vi "Find Average Center.vi"(5 "Position":i32, 7 "Tray Number":i32, 8 "Assembly Type":string, 9 "XYZTheta":dbl[](array[numeric]), 10 "Sensor Thickness":dbl, 11 "Gantry In":refnum<k24>) -> (1 "XYZTheta":dbl[](array[numeric]) format="%.6g", 3 "Gantry Out":refnum<k24>)   [LabVIEW 2021, in "Component Tray.lvclass"]
uses:
  Component Tray.lvclass
  Find Component.ctl
  Controller/Camera/Machine Vision.ctl
  C:/Program Files (x86)/Aerotech/A3200/LabVIEW/2010/Bin/Aerotech.A3200.dll
  Program Files (x86)/Aerotech/A3200/LabVIEW/2010/Bin/Aerotech.A3200.dll
  Controller/Camera/Camera settings.ctl
  <vilib>/vision/Pattern Matching.llb/IMAQ Pattern Match Advanced Options.ctl
  Controller/Camera/Edmund Optics/Edmund Optics.lvclass
  C:/Users/HEP/Documents/GitHub/Gantry/UCSB-Gantry-HEP-main/Classes/Controller/Camera/Camera.lvclass
  Controller/Camera/Camera.lvclass
  Controller/Motion/A3200/A3200.lvclass
  Controller/Motion/Motion.lvclass
  <vilib>/vision/NI_Vision_Development_Module.lvlib
  <vilib>/vision/Image Controls.llb/IMAQ Image.ctl
panel:
  in  "Algorithm":i32(ring)=2 items=["All", "Low Discrepancy Sampling", "Grayscale Value Pyramid", "Gradients Pyramid"]
  in  "Parameters":T1={"Number of Matches Requested"=1, "Minimum Match Score"=800.0, "Angle Ranges"=[]}
  in  "ROI Descriptor":T2 {"Contours"."Type" items=["No Selection", "Point", "Line", "Rectangle", "Oval", "Polygon", "Freehand Region", "Annulus", "Unused2", "Unused3", "Broken Line", "Freehand Line", "Rotated Rectangle"]}
  in  "Advanced Options":cluster{"Item":T3, "Value":dbl}[](array[cluster]) {"Item" items=["LD Sampling - Minimum Constrast"=0, "LD Sampling - Enable Subpixel Accuracy"=1, "LD Sampling - Search Strategy"=2, "LD Sampling - Subpixel Iterations"=3, "LD Sampling - Subpixel Tolerance"=4, "LD Sampling - Initial Match List Length"=5, "LD Sampling - Match List Reduction Factor"=6, "LD Sampling - Initial Step Size"=7, "LD Sampling - Intermediate Angular Accuracy"=8, "-"=9, "Pyramid - Max Pyramid Level"=100, "Pyramid - Minimum Contrast"=102, "Pyramid - Enable Subpixel Accuracy"=103, "Pyramid - Subpixel Iterations"=104, "Pyramid - Subpixel Tolerance"=105, "Pyramid - Initial Match List Length"=106, "Pyramid - Match List Reduction Factor"=107, "Pyramid - Intermediate Angular Accuracy"=108, "Pyramid - Process Border Matches"=109, "Pyramid - Min Match Separation Distance"=111, "Pyramid - Min Match Separation Angle"=112, "Pyramid - Max Match Overlap"=113, "Pyramid - Max Cache in MB"=114, "Pyramid - Clear Cache"=115, "Pyramid - Enable Accurate Score Computation"=116, "Pyramid - Interpolation Method For Score Computation"=117, "Pyramid - Enable Target To Template Score"=118, "-"=119, "Enable Defect Map"=200]}
  out "Array":i32[](array[numeric])
  out "Checking Sensor ID":bool
  out "All Matches XY":sgl[][](array[numeric])
  out "Match found?":bool
  in  "Focus":bool
  out "Gantry":dbl[](array[numeric]) format="%.6g"
  out "Sum":dbl[](array[numeric]) format="%.6g"
  in  "Machine Vision":T4
  out "Radius (Real-World)":dbl
  out "Standard Variation":sgl
  out "Maximal Value":sgl
  out "Average Strength":dbl
  out "Instructions":string
  out "Camera":dbl[](array[numeric])
  out "Image":T5(plugin-control)
  in  "Enter Manual Mode":bool
  out "Manual Mode On":bool
  in  "Auto Submit":bool
  out "Tray and Position":string
  out "Sensor ID":picture[](array[picture])
  out "Sensor ID":string
  out "predicted fiducials":dbl[][](array[numeric])
  out "Current Z High Speed":dbl
  out "Current XY High Speed":dbl
  out "current Z low speed":dbl
  out "current XY speed":dbl
  in  "Z high":dbl=12.5
  in  "XY high":dbl=50.0
  in  "Z low":dbl=0.05
  in  "XY low":dbl=0.1
  in  "Predict fiducials":bool
  out "Low Speed":bool
  out "X":bool
  out "Y":bool
  out "Z":bool
  out "High Speed":bool
  in  "Go to CH191/FD5":bool
  in  "Go to CH197/FD4":bool
  out "Program Done?":bool
  out "Sensor ID Location":dbl[](array[numeric])
  in  "Go to Sensor ID":bool
  out "CH1 XYZ":dbl[](array[numeric])
  out "CH1 correct?":bool
  in  "Go to CH1":bool
  out "All fiducials recorded":bool
  in  "Override camera presets":bool
  in  "Camera settings":T6={"Gamma"=1.6, "Gain"=0, "Sharpness"=0, "Contrast"=0.0, "Exposure"=0.0078125} {"Exposure" min=0.000244140625 max=0.5 scale=0.0002..0.5; "Contrast" min=0.0 max=1.0 scale=0.001..1.0; "Sharpness" min=0 max=2 step=1 scale=0.0..2.0; "Gain" min=0 max=100 step=1 scale=0.1..100.0; "Gamma" min=0.01 max=10.0 scale=0.01..10.0}
  out "CH197/FD4 XYZ":dbl[](array[numeric]) format="%.6g"
  out "CH8/FD2 XYZ":dbl[](array[numeric]) format="%.6g"
  out "CH191/FD5 XYZ":dbl[](array[numeric]) format="%.6g"
  out "CH1/FD1 XYZ":dbl[](array[numeric]) format="%.6g"
  in  "Record CH8/FD2":bool
  in  "Record CH197/FD4":bool
  in  "Record CH191/FD5":bool
  in  "Record CH1/FD1":bool
  in  "Go to CH8/FD2":bool
  in  "Go to CH1/FD1":bool
  in  "Joystick":bool
  in  "Go to Center":bool
  in  "Component":T7
  in  "Stop Program":bool
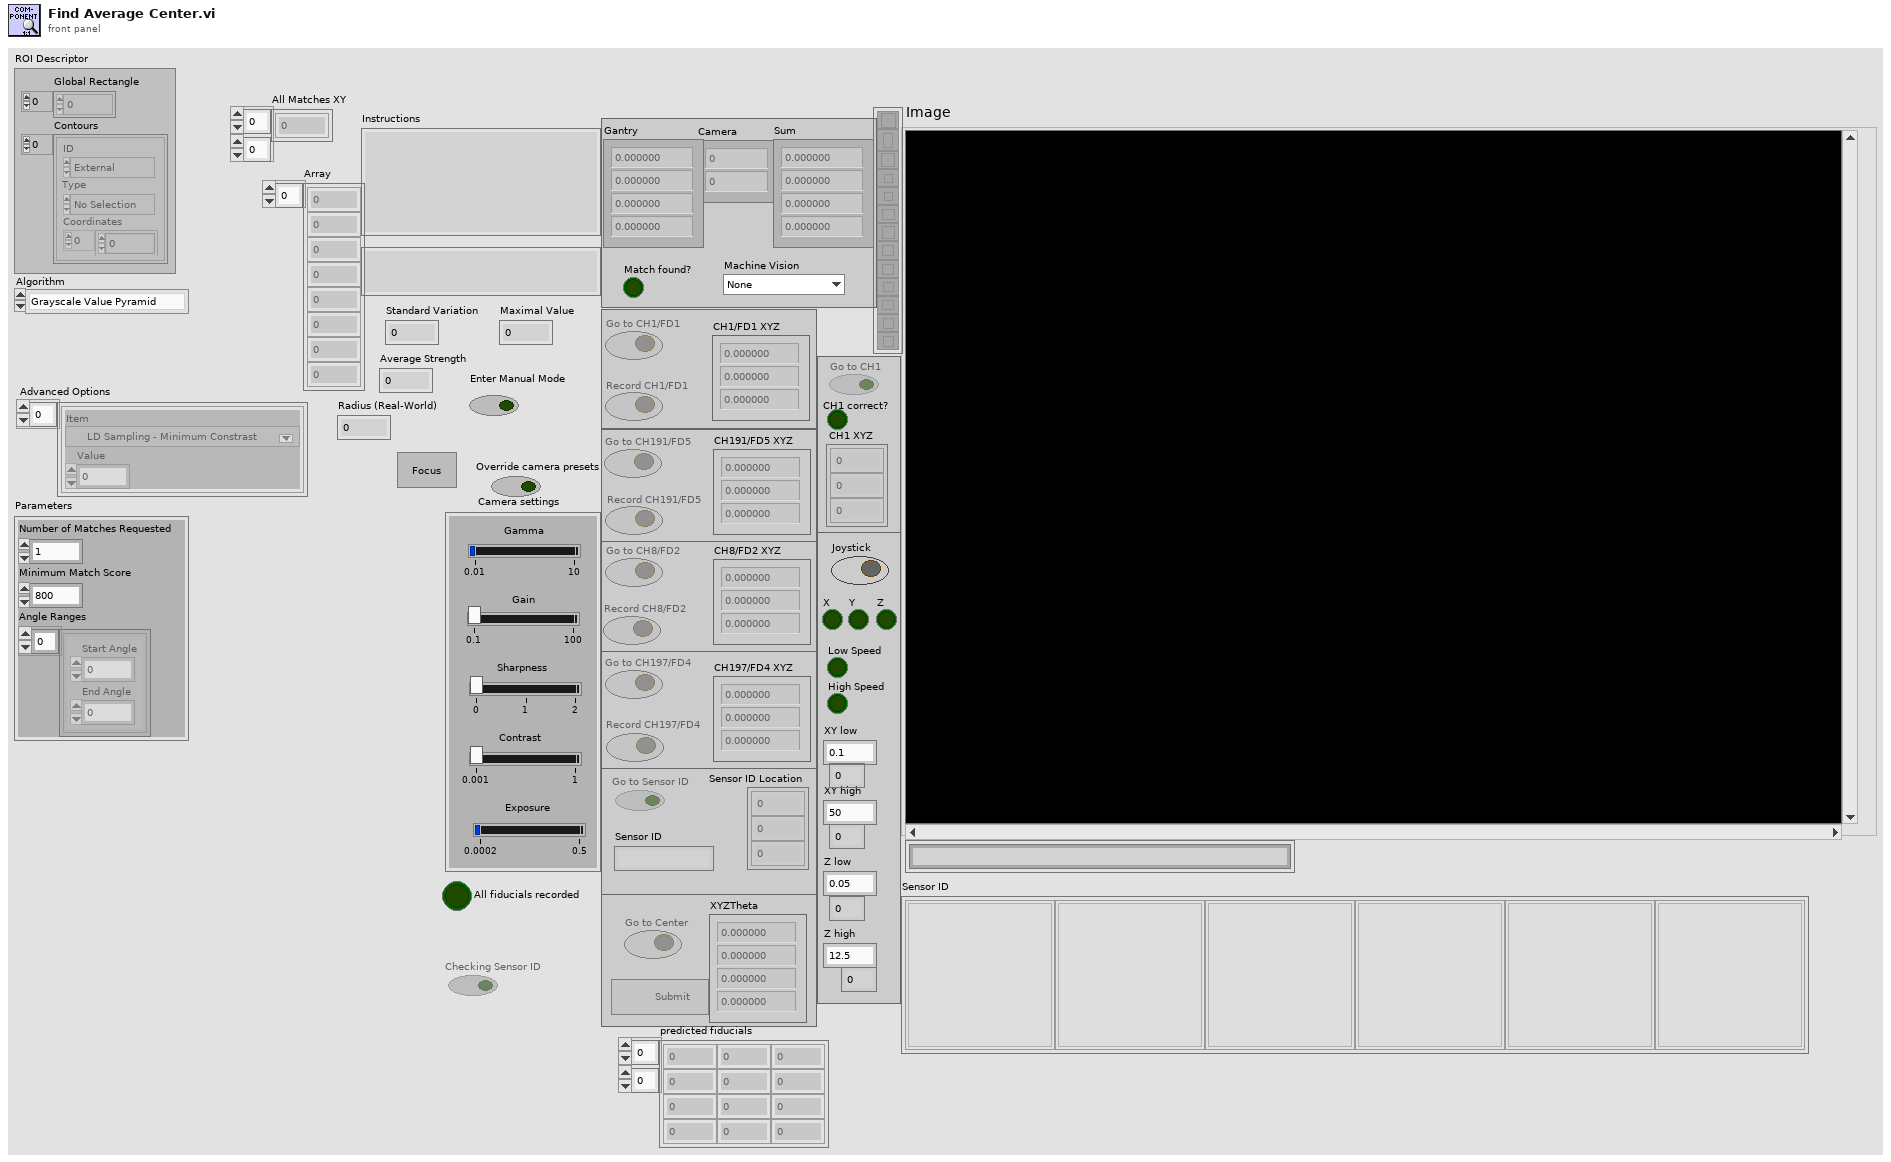
[diagram p1: front panel]
types:
  T1 = cluster{"Number of Matches Requested":i32, "Minimum Match Score":sgl, "Angle Ranges":cluster{"Start Angle":sgl, "End Angle":sgl}[]}
  T2 = typedef "ROI Descriptor" = cluster{"Global Rectangle":i32[], "Contours":cluster{"ID":enum32{"External", "Internal"}, "Type":u32, "Coordinates":i32[]}[]}
  T3 = typedef "IMAQ Pattern Match Advanced Options.ctl" = u16
  T4 = typedef "Camera.lvclass/Machine Vision.ctl" = enum16{"None", "Assembly Tray Circle", "Assembly Tray Fiducial", "Partial Hexaboard", "sensor edge init", "HB edge init", "sensor edge pos1", "sensor edge pos2", "HB edge pos1", "HB edge pos2", "Sensor CH1-2", "HB CH1", "HB CH2", "V3 Sensor Circle", "Hexaboard Circle", "sensor CH1 check", "HB CH1 check ", "sensor ID"}
  T5 = typedef "IMAQ Image.ctl" = refnum<image>
  T6 = typedef "Camera.lvclass/Camera settings.ctl" = cluster{"Gamma":dbl, "Gain":i64, "Sharpness":i64, "Contrast":dbl, "Exposure":dbl}
  T7 = typedef "Component Tray.lvclass/Find Component.ctl" = cluster{"New Fiducials":dbl[], "Past Fiducials":dbl[][], "XYZTheta":dbl[], "Fiducials Path":path, "Position":i32, "CH1 Location":dbl[], "Sensor ID Location":dbl[], "initial rotation":dbl[], "CH2 location":dbl[], "max std variation":dbl, "max strength":dbl, "CH2 pattern matching":T4, "Fiducial Circle":T4, "Get Edge":T4, "Pos multiplier":dbl, "time to wait":u32, "fiducial to edge":dbl, "Protomodule?":bool, "Assembly Type":string, "CH1 to CH2":dbl, "Tray Number":string, "fiducial radius":dbl, "4 fiducials?":bool, "CH1 check":T4, "Edge Scan":T4, "CH1 pattern matching":T4, "Sensor Thickness":dbl, "Previous Avgs":dbl[][], "avg value count":dbl[]}
  T8 = enum8{"Enabled", "Disabled", "Disabled and Grayed Out"}
  T9 = enum16{"None", "Assembly Tray Circle", "Assembly Tray Fiducial", "Partial Hexaboard", "sensor edge init", "HB edge init", "sensor edge pos1", "sensor edge pos2", "HB edge pos1", "HB edge pos2", "Sensor CH1-2", "HB CH1", "HB CH2", "V3 Sensor Circle", "Hexaboard Circle", "sensor CH1 check", "HB CH1 check "}
  T10 = cluster{"Average Strength":dbl, "Radius (Real-World)":dbl, "Match found?":bool, "initial angle":sgl, "Global Report":cluster{"Mean Value":sgl, "Standard Variation":sgl, "Minimal Value":sgl, "Maximal Value":sgl, "Area (calibrated)":sgl, "Area (pixels)":u32, "%":sgl, "Calibration Valid":bool}}
  T11 = typedef "IMAQ GM Match Report.ctl" = cluster{"Position":cluster{"x":sgl, "y":sgl}, "Angle":sgl, "Scale":sgl, "Score":sgl, "Bounding Box":cluster{"x":sgl, "y":sgl}[], "Contrast Reversed":bool, "Occlusion %":sgl, "Template Target Curve Score":sgl, "Target Template Curve Score":sgl, "Correlation Score":sgl}
  T12 = cluster{"Mean Value":sgl, "Standard Variation":sgl, "Minimal Value":sgl, "Maximal Value":sgl, "Area (calibrated)":sgl, "Area (pixels)":u32, "%":sgl, "Calibration Valid":bool}
  T13 = cluster{"left":i16, "top":i16, "right":i16, "bottom":i16}
  T14 = typedef "File Paths.ctl" = cluster{"Glue Pattern Folder":path, "Carrier Tray Folder":path, "Pick Up Tool Fixture Folder":path, "Components Folder":path, "Bellows Tool Offset.txt":path, "Pick Up Tool Offset.txt":path, "Dispense Tip Offset.txt":path, "Log Files":path, "Gantry Assembly Map.txt":path, "Syringe and offset map.txt":path, "Controllers Folder":path, "Local dbase config":path}
  T15 = typedef "imagedata.ctl" = cluster{"image type":i32, "image depth":i32, "image":u8[], "mask":u8[], "colors":u32[], "Rectangle":cluster{"left":i16, "top":i16, "right":i16, "bottom":i16}}
  T16 = cluster{"left":dbl, "top":dbl, "right":dbl, "bottom":dbl}
  T17 = cluster{"Position":cluster{"x":sgl, "y":sgl}, "Angle":sgl, "Scale":sgl, "Score":sgl, "Bounding Box":cluster{"x":sgl, "y":sgl}[]}[]
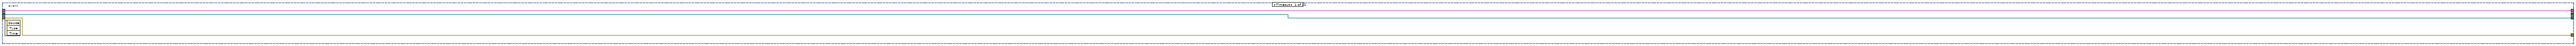
[diagram p3: hidden frame]
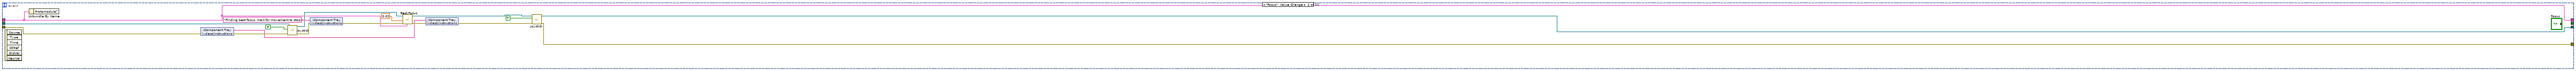
[diagram p4: hidden frame]
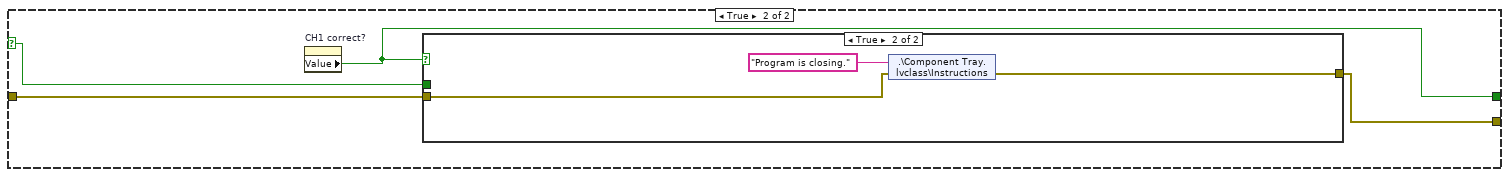
[diagram p5: hidden frame]
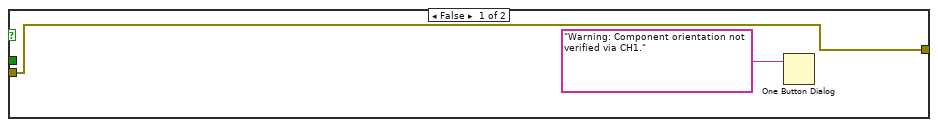
[diagram p6: hidden frame]
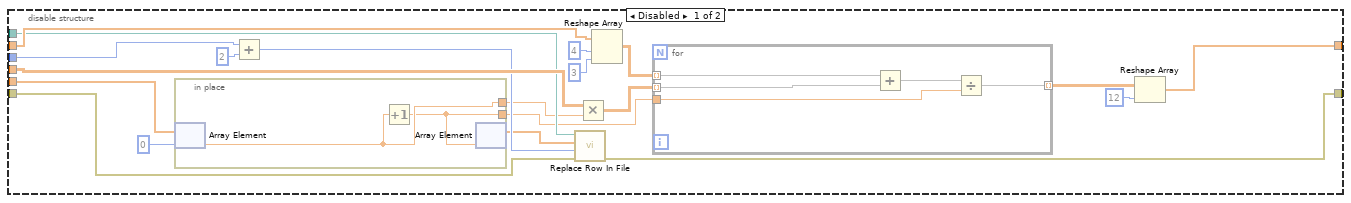
[diagram p8: hidden frame]
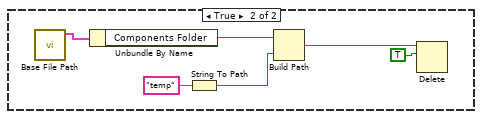
[diagram p9: hidden frame]
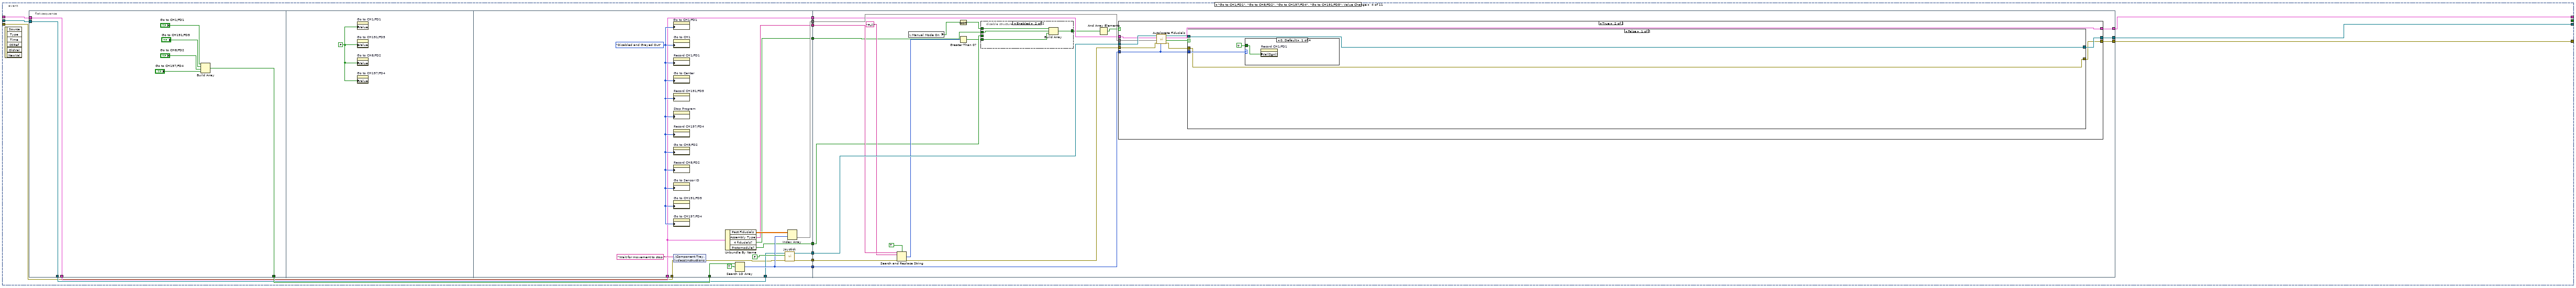
[diagram p10: hidden frame]
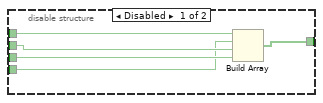
[diagram p11: hidden frame]
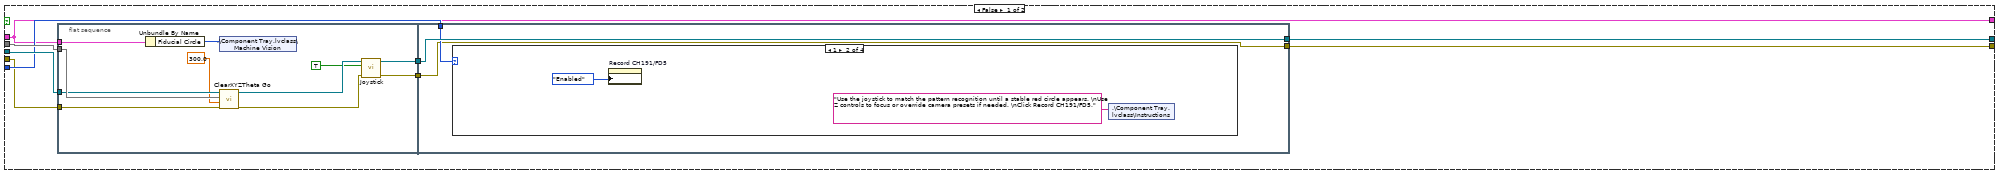
[diagram p12: hidden frame]
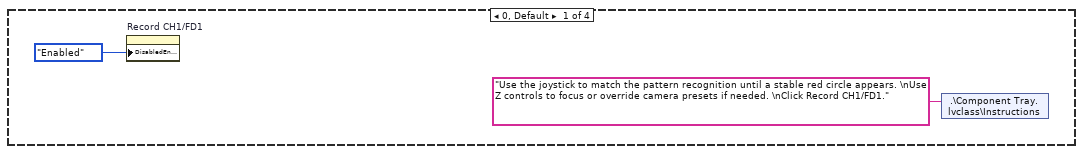
[diagram p13: hidden frame]
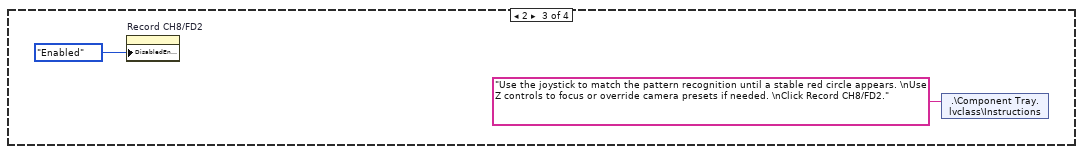
[diagram p14: hidden frame]
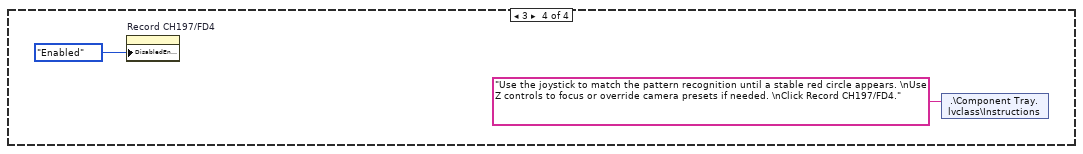
[diagram p15: hidden frame]
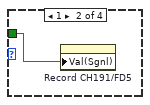
[diagram p16: hidden frame]
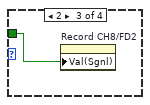
[diagram p17: hidden frame]
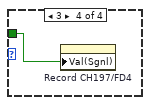
[diagram p18: hidden frame]
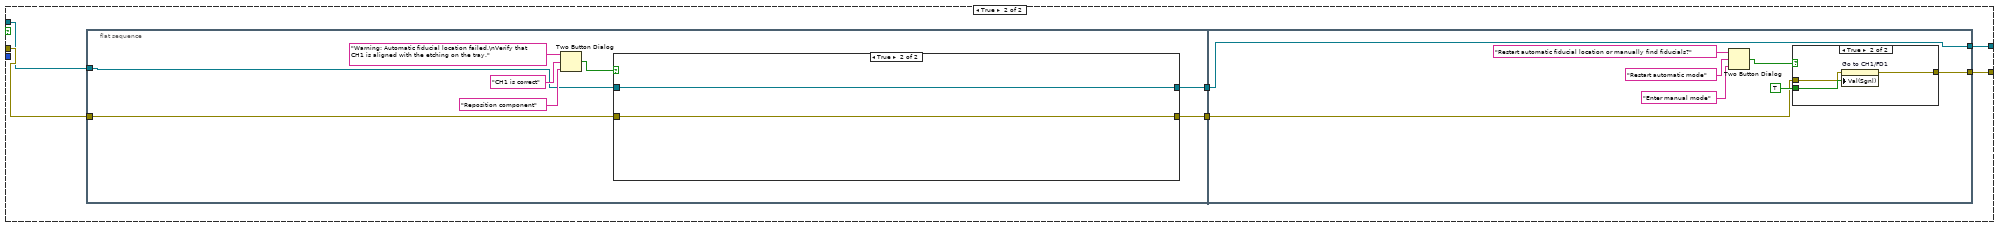
[diagram p19: hidden frame]
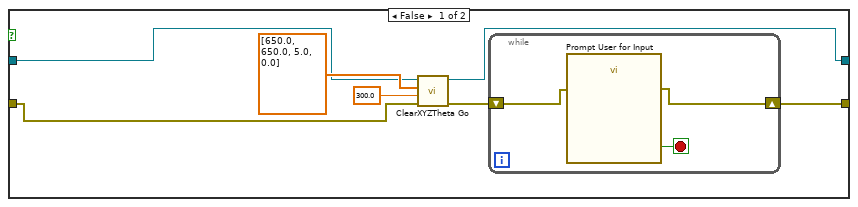
[diagram p20: hidden frame]
diagram:
  n1 = flat-sequence {
    tunnel: [w20] -> w13
    tunnel: [w22] -> w11
    tunnel: ["Gantry In"] -> w9
    tunnel: ["Position"] -> w8
    tunnel: [w28] -> w6
    tunnel: w13 -> [w28]
    tunnel: [w27] -> w5
    tunnel: w11 -> [w27]
    tunnel: [w26] -> w4
    tunnel: w9 -> [w26]
    tunnel: [w25] -> w3
    tunnel: w8 -> [w25]
    tunnel: [w24] -> w1
    tunnel: [w34] -> w12
    tunnel: w6 -> [w34]
    tunnel: w5 -> [w37]
    tunnel: [w37] -> w10
    tunnel: [w36] -> w2
    tunnel: w4 -> [w36]
    tunnel: [w35] -> w7
    tunnel: w3 -> [w35]
    frame #0 {
      w22 = refnum<class "Edmund Optics.lvclass"> refnum  # Edmund Optics.lvclass
      (unwired) 1 ("y")
      n2 = call "Find Average Center Setup.vi"("Sensor Thickness"="Sensor Thickness", "Assembly Type"="Assembly Type", "Position"="Position", "Tray Number"="Tray Number", "XYZTheta"="XYZTheta", "Component"="Component") -> ("output cluster"=w20:T7)  [unwired: 5 in]
    }
    frame #1 {
      n3 = control-ref of="This VI"() -> (w29:refnum<vi>)
      n4 = invoke class="VI" method="Default Vals.Reinit All"(reference=w29) -> (error out=w24:errorcluster)  [unwired: 2 in, 2 out]
    }
    frame #2 {
      n5 = Unbundle By Name(w34) -> ("4 fiducials?"=w30:bool)
      n6 = Select(t=T8."Enabled" ("Disabled"), s=w30, f=T8."Disabled and Grayed Out" ("Disabled")) -> (s? t:f=w31:T8)
      n7 = property on="CH197/FD4 XYZ" class="Arr (strict)"("DisabledEnum"=w31) -> ()  [unwired: 2 in, 2 out]
      n8 = property on="Record CH191/FD5" class="Bool (strict)"("DisabledEnum"=w31) -> ()  [unwired: 2 in, 2 out]
      n9 = property on="Predict fiducials" class="Bool (strict)"("DisabledEnum"=w31) -> ()  [unwired: 2 in, 2 out]
      n10 = property on="Record CH197/FD4" class="Bool (strict)"("DisabledEnum"=w31) -> ()  [unwired: 2 in, 2 out]
      n11 = property on="Go to CH197/FD4" class="Bool (strict)"("DisabledEnum"=w31) -> ()  [unwired: 2 in, 2 out]
      n12 = property on="CH191/FD5 XYZ" class="Arr (strict)"("DisabledEnum"=w31) -> ()  [unwired: 2 in, 2 out]
      n13 = property on="Go to CH191/FD5" class="Bool (strict)"("DisabledEnum"=w31) -> ()  [unwired: 2 in, 2 out]
    }
  }
  n14 = while {
    shift-right: [w62] -> _
    shift-left: w10 -> [w64]
    shift-right: [w45] -> _
    shift-left: w2 -> [w47]
    i -> [w59]
    stop <- w43 stop-if-true
    n15 = in-place {
      in-place-border: [w90] -> w46
      in-place-border: w47 -> [w72]
      # "Joystck Status"
      n16 = call "Get Joytick Status.vi"("Gantry In"=w72) -> ("JoystickLowSpeedActive"=w94:bool, "Joystick Status"=w95:bool[], "Gantry Out"=w91:refnum<k24>, "High Speeds"=w79:dbl[], "Low Speeds"=w78:dbl[])  [unwired: 5 in, 1 out]
      n17 = Build Array("XY low", "XY low", "XY low", "Z low") -> (w85:dbl[])
      n18 = Build Array("XY high", "XY high", "XY high", "Z high") -> (w84:dbl[])
      n19 = call "Set Joystick Speed.vi"("High Speed Inputs"=w84, "Low Speed Inputs"=w85, "Gantry"=w91) -> ("Controller Out"=w90:refnum<k24>)  [unwired: 7 in, 1 out]
      n20 = Or Array Elements(Boolean array=w95) -> (logical OR=w92:bool)
      n21 = Not(x=w94) -> (.not. x?=w93:bool)
      n22 = Index Array(array=w79) -> (element #1=→"Current XY High Speed":dbl, element #3=→"Current Z High Speed":dbl)  [unwired: 3 in, 1 out]
      n23 = Index Array(array=w78) -> (element #1=→"current XY speed":dbl, element #3=→"current Z low speed":dbl)  [unwired: 3 in, 1 out]
      n24 = Index Array(array=w95) -> (element #1=→"X":bool, element #2=→"Y":bool, element #3=→"Z":bool)  [unwired: 3 in]
      n25 = And(x=w93, y=w92) -> (x .and. y?=→"High Speed":bool)
      n26 = And(x=w92, y=w94) -> (x .and. y?=→"Low Speed":bool)
    }
    n27 = local read "Checking Sensor ID"() -> (w38:bool)
    n28 = shared-variable ".\\Component Tray.lvclass\\Instructions"() -> (→"Instructions":string)  [unwired: 1 in, 1 out]
    n29 = property on="Manual Mode On" class="Bool (strict)"() -> ("Value"=w40:bool)  [unwired: 2 in, 2 out]
    n30 = shared-variable ".\\Component Tray.lvclass\\Manual Mode"("Enter Manual Mode") -> ()  [unwired: 1 in, 1 out]
    n31 = Or(x=w40, y=w38) -> (x .or. y?=w39:bool)
    n32 = case shown="True" w39 {
      tunnel: [w96 "Machine Vision"] -> w48
      frame False {
        n33 = shared-variable ".\\Component Tray.lvclass\\Machine Vision"() -> (w96:T9)  [unwired: 1 in, 1 out]
      }
      frame True {
      }
    }
    n34 = local read "Program Done?"() -> (w43:bool)
    n35 = Equal To 0?(x=w59) -> (x = 0?=w58:bool)
    n36 = call "Camera.vi"("Camera in"=w64, "Stop"=w43, "Machine Vision"=w48, "Camera settings"="Camera settings", "Loop 0"=w58, "Override presets"="Override camera presets") -> ("All Matches XY"=→"All Matches XY":sgl[][], "Camera out"=w62:refnum<class "Edmund Optics.lvclass">, "output cluster"=w57:T10, "pattern matching"=w50:T11, "Image"=→"Image":T5, "Camera"=w42:dbl[])  [unwired: 6 in, 2 out]
    "Camera" <- w42
    n37 = Unbundle By Name(w57) -> ("Average Strength"=w56:dbl, "Radius (Real-World)"=w55:dbl, "Match found?"=w54:bool, "Global Report"=w53:T12)
    "Average Strength" <- w56
    "Radius (Real-World)" <- w55
    "Match found?" <- w54
    n38 = shared-variable ".\\Component Tray.lvclass\\pattern matching"(w50) -> ()  [unwired: 1 in, 1 out]
    n39 = shared-variable ".\\Component Tray.lvclass\\Camera"(w42) -> ()  [unwired: 1 in, 1 out]
    n40 = in-place {
      in-place-border: w46 -> [w67]
      in-place-border: [w66] -> w45
      in-place-border: w42 -> [w65]
      # "Current Position"
      n41 = call "Get Current Position.vi"("Gantry In"=w67) -> ("XYZTheta Out"=w70:dbl[], "Gantry Out"=w66:refnum<k24>)  [unwired: 8 in, 1 out]
      "Gantry" <- w70
      n42 = Reshape Array(w65, 4 ("dimension size")) -> (w69:dbl[])
      n43 = Add(x=w70, y=w69) -> (x+y=→"Sum":dbl[])
    }
    n44 = shared-variable ".\\Component Tray.lvclass\\Average Strength"(w56) -> ()  [unwired: 1 in, 1 out]
    n45 = shared-variable ".\\Component Tray.lvclass\\Radius (Real-World)"(w55) -> ()  [unwired: 1 in, 1 out]
    n46 = shared-variable ".\\Component Tray.lvclass\\Match found?"(w54) -> ()  [unwired: 1 in, 1 out]
    n47 = Unbundle By Name(w53) -> ("Standard Variation"=w52:sgl, "Maximal Value"=w51:sgl)
    "Maximal Value" <- w51
    "Standard Variation" <- w52
    n48 = shared-variable ".\\Component Tray.lvclass\\Standard Variation"(w52) -> ()  [unwired: 1 in, 1 out]
    n49 = shared-variable ".\\Component Tray.lvclass\\Maximal Value"(w51) -> ()  [unwired: 1 in, 1 out]
  }
  n50 = while {
    shift-right: [w107] -> _
    shift-left: w12 -> [w100]
    shift-right: [w105] -> w14
    shift-left: w2 -> [w106]
    tunnel: w7 -> [w101]
    shift-right: [w98] -> _
    shift-left: w1 -> [w99]
    i -> [w104]
    stop <- w108 stop-if-true
    n51 = event shown="[2] \"Stop Program\", \"Auto Submit\": Value Change" {
      selector: _ -> [_ _ _ _ _ _ _ _ _ _ _]
      dyn-events: _ -> [_ _ _ _ _ _ _ _ _ _ _]
      timeout: _ -> [_ _ _ _ _ _ _ _ _ _ _]
      tunnel: [_ _ w147 _ _ _ _ _ _ _ _] -> w108
      tunnel: w100 -> [w126 w127 w151 w233 w384 w464 w491 w499 w541 w669 w689]
      tunnel: [w126 w127 w151 w229 w391 w463 w491 w499 w541 w669 w689] -> w107
      tunnel: w106 -> [w125 w134 w152 w237 w407 w468 w490 w498 w547 w671 w688]
      tunnel: [w125 w131 w150 w231 w385 w468 w488 w496 w545 w671 w687] -> w105
      tunnel: w99 -> [w124 w138 w144 w223 w390 w461 w487 w494 w537 w666 w685]
      tunnel: [w124 w128 w145 w221 w388 w461 w486 w492 w535 w666 w684] -> w98
      event Timeout {
        n52 = event-data() -> ()  [unwired: 1 in, 3 out]
      }
      event "Focus": Value Change {
        n53 = event-data() -> ()  [unwired: 1 in, 6 out]
        n54 = Unbundle By Name(w127) -> ()  [unwired: 1 out]
        n55 = shared-variable ".\\Component Tray.lvclass\\Instructions"(error in=w138) -> (w140:string, error out=w136:errorcluster)
        n56 = call "Joystick.vi"("error in (no error)"=w136, "Joystick"=FALSE, "Gantry In"=w134) -> ("error out"=w135:errorcluster, "Gantry Out"=w133:refnum<k24>)  [unwired: 7 in]
        n57 = shared-variable ".\\Component Tray.lvclass\\Instructions"("Finding best focus. Wait for movement to stop." ("Instructions"), error in=w135) -> (error out=w142:errorcluster)
        n58 = call "Best Focus.vi"("Component"=w127, "error in (no error)"=w142, "Inc by"=0.02, "Gantry In"=w133) -> ("error out"=w141:errorcluster, "Gantry Out"=w130:refnum<k24>)  [unwired: 4 in, 2 out]
        n59 = shared-variable ".\\Component Tray.lvclass\\Instructions"(w140, error in=w141) -> (error out=w129:errorcluster)
        n60 = call "Joystick.vi"("error in (no error)"=w129, "Joystick"=TRUE, "Gantry In"=w130) -> ("error out"=w128:errorcluster, "Gantry Out"=w131:refnum<k24>)  [unwired: 7 in]
      }
      event "Stop Program", "Auto Submit": Value Change {
        n61 = event-data() -> ()  [unwired: 1 in, 6 out]
        n62 = flat-sequence {
          frame #0 {
          }
          frame #1 {
            n63 = property on="Auto Submit" class="Bool (strict)"("Value"=FALSE ("Auto Submit")) -> ()  [unwired: 2 in, 2 out]
          }
        }
        n64 = property on="All fiducials recorded" class="Bool (strict)"() -> ("Value"=w149:bool)  [unwired: 2 in, 2 out]
        n65 = case shown="False" w149 {
          selector: w149 -> [w154 w159]
          tunnel: [w154 w158] -> w148
          tunnel: [w153 w157] -> w146
          tunnel: w144 -> [w153 w156]
          frame False {
            n66 = One Button Dialog(message="Warning: At least one fiducial not recorded.") -> ()  [unwired: 1 in, 1 out]
          }
          frame True {
            n67 = property on="CH1 correct?" class="Bool (strict)"() -> ("Value"=w158:bool)  [unwired: 2 in, 2 out]
            n68 = case shown="True" w158 {
              tunnel: w159 -> [_ _]
              tunnel: w156 -> [w160 w163]
              tunnel: [w160 w162] -> w157
              frame False {
                n69 = One Button Dialog(message="Warning: Component orientation not verified via CH1.") -> ()  [unwired: 1 in, 1 out]
              }
              frame True {
                n70 = shared-variable ".\\Component Tray.lvclass\\Instructions"("Program is closing." ("Instructions"), error in=w163) -> (error out=w162:errorcluster)
              }
            }
          }
        }
        n71 = case shown="True" w148 {
          selector: w148 -> [w167 w185]
          tunnel: w152 -> [w168 w184]
          tunnel: w151 -> [_ w182]
          tunnel: [w168 w183] -> w150
          tunnel: [w167 w185] -> w147
          tunnel: w146 -> [w166 w173]
          tunnel: [w166 w170] -> w145
          frame False {
          }
          frame True {
            n72 = Unbundle By Name(w182) -> ("Fiducials Path"=w175:path, "New Fiducials"=w177:dbl[], "Position"=w174:i32, "Protomodule?"=w181:bool, "Previous Avgs"=w178:dbl[][], "avg value count"=w169:dbl[])
            n73 = call "Joystick.vi"("error in (no error)"=w173, "Joystick"=FALSE, "Gantry In"=w184) -> ("error out"=w172:errorcluster, "Gantry Out"=w183:refnum<k24>)  [unwired: 7 in]
            n74 = case shown="False" w181 {
              frame False {
              }
              frame True {
                n75 = call "Base File Path.vi"() -> ("Paths Out"=w219:T14)  [unwired: 11 in]
                n76 = Unbundle By Name(w219) -> ("Components Folder"=w217:path)
                n77 = String To Path(string="temp") -> (path=w218:path)
                n78 = Build Path(base path=w217, name or relative path=w218) -> (appended path=w220:path)
                n79 = Delete(path (use dialog)=w220, entire hierarchy (F)=TRUE) -> ()  [unwired: 3 in, 3 out]
              }
            }
            n80 = disable-structure shown="Enabled" {
              disable-tunnel: w178 -> [w205 _]
              disable-tunnel: w177 -> [w198 w214]
              disable-tunnel: [w197 w214] -> w176
              disable-tunnel: w175 -> [w196 _]
              disable-tunnel: w174 -> [w195 _]
              disable-tunnel: w172 -> [w192 w213]
              disable-tunnel: [w191 w213] -> w171
              disable-tunnel: w169 -> [w190 _]
              frame Disabled {
                n81 = in-place {
                  in-place-border: [w207] -> w188
                  in-place-border: [w206] -> w187
                  n82 = in-place-array #1(w190, 0) -> (w207:dbl)
                  n83 = Increment(x=w207) -> (x+1=w206:dbl)
                  n84 = in-place-array #1(w206) -> (w189:dbl[])  [unwired: 1 out]
                }
                n85 = Add(x=w195, y=2) -> (x+y=w193:i32)
                n86 = call "Replace Row In File.vi"("error in"=w192, "Index"=w193, "Insert Array"=w189, "Path"=w196) -> ("error out"=w191:errorcluster)  [unwired: 7 in]
                n87 = Multiply(x=w205, y=w188) -> (x*y=w201:dbl[][])
                n88 = Reshape Array(w198, 4 ("dimension size"), 3 ("dimension size")) -> (w202:dbl[][])
                n89 = for {
                  tunnel: w202 -> [w212] mode=indexing
                  tunnel: w201 -> [w211] mode=indexing
                  tunnel: w187 -> [w209]
                  tunnel: [w208] -> w200 mode=indexing
                  n90 = Add(x=w212, y=w211) -> (x+y=w210:dbl[])
                  n91 = Divide(x=w210, y=w209) -> (x/y=w208:dbl[])
                }
                n92 = Reshape Array(w200, 12 ("dimension size")) -> (w197:dbl[])
              }
              frame Enabled {
              }
            }
            n93 = shared-variable ".\\Component Tray.lvclass\\Instructions"("Program is done." ("Instructions")) -> ()  [unwired: 1 in, 1 out]
            n94 = call "Replace Row In File.vi"("error in"=w171, "Index"=w174, "Insert Array"=w176, "Path"=w175) -> ("error out"=w170:errorcluster)  [unwired: 7 in]
          }
        }
        "Program Done?" <- w147
      }
      event "Go to CH1/FD1", "Go to CH8/FD2", "Go to CH197/FD4", "Go to CH191/FD5": Value Change {
        n95 = event-data() -> ()  [unwired: 1 in, 6 out]
        n96 = flat-sequence {
          tunnel: w237 -> [w239]
          tunnel: w233 -> [w238]
          tunnel: [w240] -> w226
          tunnel: [w239] -> w225
          tunnel: [w238] -> w224
          tunnel: [w259] -> w236
          tunnel: [w257] -> w234
          tunnel: [w260] -> w235
          tunnel: [w255] -> w232
          tunnel: [w249] -> w230
          tunnel: [w254] -> w228
          tunnel: [w252] -> w227
          tunnel: w226 -> [w251]
          tunnel: w225 -> [w250]
          tunnel: w224 -> [w249]
          tunnel: w223 -> [w248]
          tunnel: [w246] -> w222
          tunnel: w236 -> [w282]
          tunnel: w235 -> [w281]
          tunnel: w234 -> [w276]
          tunnel: w232 -> [w280]
          tunnel: [w275] -> w231
          tunnel: w230 -> [w274]
          tunnel: [w273] -> w229
          tunnel: w228 -> [w271]
          tunnel: w227 -> [w269]
          tunnel: w222 -> [w265]
          tunnel: [w263] -> w221
          frame #0 {
            n97 = Build Array "Build Array"("Go to CH1/FD1", "Go to CH191/FD5", "Go to CH8/FD2", "Go to CH197/FD4") -> (w240:bool[])
          }
          frame #1 {
            w245 = FALSE ("Go to Top Right Fiducial")
            n98 = property on="Go to CH1/FD1" class="Bool (strict)"("Value"=w245) -> ()  [unwired: 2 in, 2 out]
            n99 = property on="Go to CH191/FD5" class="Bool (strict)"("Value"=w245) -> ()  [unwired: 2 in, 2 out]
            n100 = property on="Go to CH8/FD2" class="Bool (strict)"("Value"=w245) -> ()  [unwired: 2 in, 2 out]
            n101 = property on="Go to CH197/FD4" class="Bool (strict)"("Value"=w245) -> ()  [unwired: 2 in, 2 out]
          }
          frame #2 {
            w262 = T8."Disabled and Grayed Out" ("Disabled")
            n102 = property on="Go to CH1/FD1" class="Bool (strict)"("DisabledEnum"=w262) -> ()  [unwired: 2 in, 2 out]
            n103 = property on="Go to CH1" class="Bool (strict)"("DisabledEnum"=w262) -> ()  [unwired: 2 in, 2 out]
            n104 = property on="Record CH1/FD1" class="Bool (strict)"("DisabledEnum"=w262) -> ()  [unwired: 2 in, 2 out]
            n105 = property on="Go to Center" class="Bool"("DisabledEnum"=w262) -> ()  [unwired: 2 in, 2 out]
            n106 = property on="Record CH191/FD5" class="Bool (strict)"("DisabledEnum"=w262) -> ()  [unwired: 2 in, 2 out]
            n107 = property on="Stop Program" class="Bool"("DisabledEnum"=w262) -> ()  [unwired: 2 in, 2 out]
            n108 = property on="Record CH197/FD4" class="Bool (strict)"("DisabledEnum"=w262) -> ()  [unwired: 2 in, 2 out]
            n109 = property on="Go to CH8/FD2" class="Bool (strict)"("DisabledEnum"=w262) -> ()  [unwired: 2 in, 2 out]
            n110 = property on="Record CH8/FD2" class="Bool (strict)"("DisabledEnum"=w262) -> ()  [unwired: 2 in, 2 out]
            n111 = property on="Go to Sensor ID" class="Bool (strict)"("DisabledEnum"=w262) -> ()  [unwired: 2 in, 2 out]
            n112 = property on="Go to CH191/FD5" class="Bool (strict)"("DisabledEnum"=w262) -> ()  [unwired: 2 in, 2 out]
            n113 = property on="Go to CH197/FD4" class="Bool (strict)"("DisabledEnum"=w262) -> ()  [unwired: 2 in, 2 out]
            n114 = shared-variable ".\\Component Tray.lvclass\\Instructions"("Wait for movement to stop." ("Value (Signaling)"), error in=w248) -> (error out=w247:errorcluster)
            n115 = Unbundle By Name(w249) -> ("Past Fiducials"=w256:dbl[][], "Assembly Type"=w255:string, "4 fiducials?"=w254:bool, "Protomodule?"=w252:bool)
            n116 = Search 1D Array(1D array=w251, element=TRUE) -> (index of element=w257:i32)  [unwired: 1 in]
            n117 = call "Joystick.vi"("error in (no error)"=w247, "Joystick"=FALSE, "Gantry In"=w250) -> ("error out"=w246:errorcluster, "Gantry Out"=w260:refnum<k24>)  [unwired: 7 in]
            n118 = Index Array(array=w256, index (row)=w257) -> (element=w259:dbl[])  [unwired: 1 in]
          }
          frame #3 {
            n119 = Search and Replace String(case sensitive?=TRUE ("ignore case? (F)"), input string=w280, search string="Full", error in=w265) -> (number of replacements=w277:i32, error out=w264:errorcluster)  [unwired: 4 in, 2 out]
            n120 = local read "Manual Mode On"() -> (w268:bool)
            n121 = Not(x=w268) -> (.not. x?=w267:bool)
            n122 = Greater Than 0?(x=w277) -> (x > 0?=w266:bool)
            n123 = disable-structure shown="Enabled" {
              disable-tunnel: [w287 w290] -> w272
              disable-tunnel: w271 -> [w286 w289]
              disable-tunnel: w269 -> [w285 _]
              disable-tunnel: w267 -> [w284 w291]
              disable-tunnel: w266 -> [w283 w288]
              frame Disabled {
                n124 = Build Array(w284, w283, w286, w285) -> (w287:bool[])
              }
              frame Enabled {
                n125 = Build Array(w291, w289, w288) -> (w290:bool[])
              }
            }
            n126 = And Array Elements(Boolean array=w272) -> (logical AND=w270:bool)
            n127 = case shown="True" w270 {
              tunnel: w282 -> [w300 w331]
              tunnel: w281 -> [w299 w333]
              tunnel: [w298 w327] -> w275
              tunnel: w276 -> [w295 w326]
              tunnel: w274 -> [w294 w332]
              tunnel: [w294 w330] -> w273
              tunnel: w264 -> [w293 w325]
              tunnel: [w292 w323] -> w263
              frame False {
                n128 = flat-sequence {
                  tunnel: w300 -> [w311]
                  tunnel: w299 -> [w310]
                  tunnel: [w308] -> w297
                  tunnel: [w305] -> w296
                  tunnel: w294 -> [w304]
                  tunnel: w293 -> [w301]
                  tunnel: w297 -> [w314]
                  tunnel: w296 -> [w312]
                  tunnel: w295 -> [w313]
                  tunnel: [w314] -> w298
                  tunnel: [w312] -> w292
                  frame #0 {
                    n129 = Unbundle By Name(w304) -> ("Fiducial Circle"=w303:T4)
                    n130 = shared-variable ".\\Component Tray.lvclass\\Machine Vision"(w303) -> ()  [unwired: 1 in, 1 out]
                    n131 = call "ClearXYZTheta Go.vi"("error in (no error)"=w301, "Speed"=300.0, "XYZTheta In"=w311, "Gantry In"=w310) -> ("error out"=w306:errorcluster, "Gantry Out"=w309:refnum<k24>)  [unwired: 5 in, 1 out]
                    n132 = call "Joystick.vi"("error in (no error)"=w306, "Joystick"=TRUE, "Gantry In"=w309) -> ("error out"=w305:errorcluster, "Gantry Out"=w308:refnum<k24>)  [unwired: 7 in]
                  }
                  frame #1 {
                    n133 = case shown="1" w313 {
                      frame 0, Default {
                        n134 = property on="Record CH1/FD1" class="Bool (strict)"("DisabledEnum"=T8."Enabled" ("Disabled")) -> ()  [unwired: 2 in, 2 out]
                        n135 = shared-variable ".\\Component Tray.lvclass\\Instructions"("Use the joystick to match the pattern recognition until a stable red circle appears. \nUse Z controls to focus or override camera presets if needed. \nClick Record CH1/FD1.") -> ()  [unwired: 1 in, 1 out]
                      }
                      frame 1 {
                        n136 = property on="Record CH191/FD5" class="Bool (strict)"("DisabledEnum"=T8."Enabled" ("Disabled")) -> ()  [unwired: 2 in, 2 out]
                        n137 = shared-variable ".\\Component Tray.lvclass\\Instructions"("Use the joystick to match the pattern recognition until a stable red circle appears. \nUse Z controls to focus or override camera presets if needed. \nClick Record CH191/FD5.") -> ()  [unwired: 1 in, 1 out]
                      }
                      frame 2 {
                        n138 = property on="Record CH8/FD2" class="Bool (strict)"("DisabledEnum"=T8."Enabled" ("Disabled")) -> ()  [unwired: 2 in, 2 out]
                        n139 = shared-variable ".\\Component Tray.lvclass\\Instructions"("Use the joystick to match the pattern recognition until a stable red circle appears. \nUse Z controls to focus or override camera presets if needed. \nClick Record CH8/FD2.") -> ()  [unwired: 1 in, 1 out]
                      }
                      frame 3 {
                        n140 = property on="Record CH197/FD4" class="Bool (strict)"("DisabledEnum"=T8."Enabled" ("Disabled")) -> ()  [unwired: 2 in, 2 out]
                        n141 = shared-variable ".\\Component Tray.lvclass\\Instructions"("Use the joystick to match the pattern recognition until a stable red circle appears. \nUse Z controls to focus or override camera presets if needed. \nClick Record CH197/FD4.") -> ()  [unwired: 1 in, 1 out]
                      }
                    }
                  }
                }
              }
              frame True {
                n142 = call "Autolocate Fiducials.vi"("FD Index"=w326, "error in"=w325, "Past Fiducials"=w331, "Component"=w332, "Gantry In"=w333) -> ("error out"=w324:errorcluster, "Wrong Orientation?"=w329:bool, "Component Out"=w330:T7, "Gantry Out"=w328:refnum<k24>)  [unwired: 3 in]
                n143 = case shown="False" w329 {
                  tunnel: w328 -> [w337 w346]
                  tunnel: [w337 w345] -> w327
                  tunnel: w326 -> [w336 _]
                  tunnel: w324 -> [w334 w347]
                  tunnel: [w334 w342] -> w323
                  frame False {
                    n144 = case shown="0, Default" w336 {
                      tunnel: TRUE ("Value (Signaling)") -> [w338 w339 w340 w341]
                      frame 0, Default {
                        n145 = property on="Record CH1/FD1" class="Bool (strict)"("Val(Sgnl)"=w338) -> ()  [unwired: 2 in, 2 out]
                      }
                      frame 1 {
                        n146 = property on="Record CH191/FD5" class="Bool (strict)"("Val(Sgnl)"=w339) -> ()  [unwired: 2 in, 2 out]
                      }
                      frame 2 {
                        n147 = property on="Record CH8/FD2" class="Bool (strict)"("Val(Sgnl)"=w340) -> ()  [unwired: 2 in, 2 out]
                      }
                      frame 3 {
                        n148 = property on="Record CH197/FD4" class="Bool (strict)"("Val(Sgnl)"=w341) -> ()  [unwired: 2 in, 2 out]
                      }
                    }
                  }
                  frame True {
                    n149 = flat-sequence {
                      tunnel: w347 -> [w351]
                      tunnel: w346 -> [w350]
                      tunnel: [w349] -> w344
                      tunnel: [w348] -> w343
                      tunnel: [w375] -> w345
                      tunnel: w344 -> [w375]
                      tunnel: w343 -> [w369]
                      tunnel: [w368] -> w342
                      frame #0 {
                        n150 = Two Button Dialog(message="Warning: Automatic fiducial location failed.\nVerify that CH1 is aligned with the etching on the tray.", 1:"Reposition component" ("F button name (\"Cancel\")"), 2:"CH1 is correct" ("T button name (\"OK\")")) -> (T button?=w352:bool)
                        n151 = case shown="True" w352 {
                          tunnel: w351 -> [w362 w367]
                          tunnel: w350 -> [w359 w366]
                          tunnel: [w358 w366] -> w349
                          tunnel: [w356 w367] -> w348
                          frame False {
                            n152 = call "ClearXYZTheta Go.vi"("error in (no error)"=w362, "Speed"=300.0, "XYZTheta In"=dbl[] [650.0, 650.0, 5.0, 0.0], "Gantry In"=w359) -> ("error out"=w357:errorcluster, "Gantry Out"=w358:refnum<k24>)  [unwired: 5 in, 1 out]
                            n153 = while {
                              shift-right: [w364] -> w356
                              shift-left: w357 -> [w365]
                              stop <- w363 stop-if-true
                              n154 = call "Prompt User for Input"("error in (no error)"=w365) -> ("CH1 correct?"=w363:bool, "error out"=w364:errorcluster)  [unwired: 16 in, 1 out]
                            }
                          }
                          frame True {
                          }
                        }
                      }
                      frame #1 {
                        n155 = Two Button Dialog(message="Restart automatic fiducial location or manually find fiducials?", 1:"Enter manual mode" ("F button name (\"Cancel\")"), 2:"Restart automatic mode" ("T button name (\"OK\")")) -> (T button?=w371:bool)
                        n156 = case shown="True" w371 {
                          tunnel: TRUE ("Value (Signaling)") -> [w378 w381]
                          tunnel: w369 -> [w377 w380]
                          tunnel: [w376 w379] -> w368
                          frame False {
                            n157 = property on="Enter Manual Mode" class="Bool (strict)"(error in=w377, "Val(Sgnl)"=w378) -> (error out=w376:errorcluster)  [unwired: 1 in, 1 out]
                          }
                          frame True {
                            n158 = property on="Go to CH1/FD1" class="Bool (strict)"(error in=w380, "Val(Sgnl)"=w381) -> (error out=w379:errorcluster)  [unwired: 1 in, 1 out]
                          }
                        }
                      }
                    }
                  }
                }
              }
            }
          }
        }
      }
      event "Record CH1/FD1", "Record CH191/FD5", "Record CH197/FD4", "Record CH8/FD2": Value Change {
        n159 = event-data() -> ()  [unwired: 1 in, 1 out]
        n160 = call "Get Current Position.vi"("error in (no error)"=w390, "Gantry In"=w407) -> ("error out"=w383:errorcluster, "XYZTheta Out"=w387:dbl[], "Gantry Out"=w386:refnum<k24>)  [unwired: 7 in]
        n161 = flat-sequence {
          tunnel: ["Record CH1/FD1"] -> _
          tunnel: [w430] -> w395
          frame #0 {
            n162 = Build Array "Build Array"("Record CH1/FD1", "Record CH191/FD5", "Record CH8/FD2", "Record CH197/FD4") -> (w430:bool[])
          }
          frame #1 {
            w435 = FALSE ("Record CH1/FD1")
            n163 = property on="Record CH1/FD1" class="Bool (strict)"("Value"=w435) -> ()  [unwired: 2 in, 2 out]
            n164 = property on="Record CH191/FD5" class="Bool (strict)"("Value"=w435) -> ()  [unwired: 2 in, 2 out]
            n165 = property on="Record CH197/FD4" class="Bool (strict)"("Value"=w435) -> ()  [unwired: 2 in, 2 out]
            n166 = property on="Record CH8/FD2" class="Bool (strict)"("Value"=w435) -> ()  [unwired: 2 in, 2 out]
          }
        }
        n167 = disable-structure shown="Enabled" {
          disable-tunnel: w387 -> [w419 _]
          disable-tunnel: w386 -> [w414 w429]
          disable-tunnel: [w413 w429] -> w385
          disable-tunnel: w384 -> [w412 _]
          disable-tunnel: w383 -> [w411 w428]
          disable-tunnel: [w410 w428] -> w382
          frame Disabled {
            n168 = Index Array(array=w419, index=2) -> (element=w417:dbl)
            n169 = Less?(x=w417, y=50.0) -> (x < y?=w415:bool)
            n170 = case shown="True" w415 {
              tunnel: w414 -> [w421 w427]
              tunnel: [w421 w426] -> w413
              tunnel: w412 -> [_ w425]
              tunnel: w411 -> [w420 w424]
              tunnel: [w420 w423] -> w410
              frame False {
              }
              frame True {
                n171 = call "Temp Joystick.vi"("error in (no error)"=w424, "Fiducial?"=TRUE ("Dialog?"), "Component"=w425, "Gantry In"=w427) -> ("error out"=w423:errorcluster, "Gantry Out"=w426:refnum<k24>)  [unwired: 5 in, 1 out]
              }
            }
          }
          frame Enabled {
          }
        }
        n172 = control-ref of="CH191/FD5 XYZ"() -> (w405:refnum<vi>)
        n173 = control-ref of="CH197/FD4 XYZ"() -> (w403:refnum<vi>)
        n174 = control-ref of="CH1/FD1 XYZ"() -> (w406:refnum<vi>)
        n175 = control-ref of="CH8/FD2 XYZ"() -> (w404:refnum<vi>)
        n176 = Build Array "Build Array"(w406, w405, w404, w403) -> (w409:refnum<vi>[])
        n177 = shared-variable ".\\Component Tray.lvclass\\Camera"() -> (w397:dbl[])  [unwired: 1 in, 1 out]
        n178 = Search 1D Array(1D array=w395, element=TRUE) -> (index of element=w402:i32)  [unwired: 1 in]
        n179 = Index Array "Index Array"(array=w409, index=w402) -> (element=w408:refnum<vi>)
        n180 = Reshape Array(w397, 3 ("dimension size")) -> (w396:dbl[])
        n181 = Add(x=w387, y=w396) -> (x+y=w394:dbl[])
        n182 = Multiply(x=w402, y=3) -> (x*y=w393:i32)
        n183 = property class="Arr (strict)"(reference=w408, error in=w382, "Value"=w394) -> (error out=w389:errorcluster)  [unwired: 1 out]
        n184 = property on="Manual Mode On" class="Bool (strict)"() -> ("Value"=w400:bool)  [unwired: 2 in, 2 out]
        n185 = call "Record Fiducial.vi"("CH index"=w393, "XYZ"=w394, "input cluster"=w384) -> ("All fiducials recorded"=w392:bool, "output cluster"=w391:T7)  [unwired: 7 in]
        "All fiducials recorded" <- w392
        n186 = case shown="True" w392 {
          tunnel: w400 -> [w440 w454]
          tunnel: w391 -> [w439 w453]
          tunnel: w389 -> [w437 w449]
          tunnel: [w436 w448] -> w388
          frame False {
            n187 = Unbundle By Name(w439) -> ("4 fiducials?"=w438:bool)
            n188 = case shown="False" w438 {
              selector: w438 -> [_ w447]
              tunnel: w440 -> [w442 _]
              tunnel: w437 -> [w441 w446]
              tunnel: [w441 w445] -> w436
              frame False {
                n189 = case shown="False" w442 {
                  selector: w442 -> [_ w444]
                  frame False {
                    n190 = property on="Go to CH8/FD2" class="Bool (strict)"("Val(Sgnl)"=TRUE ("Value (Signaling)")) -> ()  [unwired: 2 in, 2 out]
                  }
                  frame True {
                    n191 = property on="Enter Manual Mode" class="Bool (strict)"("Val(Sgnl)"=w444) -> ()  [unwired: 2 in, 2 out]
                  }
                }
              }
              frame True {
                n192 = property on="Predict fiducials" class="Bool (strict)"(error in=w446, "Val(Sgnl)"=w447) -> (error out=w445:errorcluster)  [unwired: 1 in, 1 out]
              }
            }
          }
          frame True {
            n193 = Unbundle By Name(w453) -> ("Sensor ID Location"=→"Sensor ID Location":dbl[], "CH1 Location"=→"CH1 XYZ":dbl[], "XYZTheta"=→"XYZTheta":dbl[])
            n194 = case shown="True" w454 {
              selector: w454 -> [_ w460]
              tunnel: w449 -> [w456 w459]
              tunnel: [w455 w458] -> w448
              frame False {
                n195 = property on="Go to CH1" class="Bool (strict)"(error in=w456, "Val(Sgnl)"=TRUE ("Value (Signaling)")) -> (error out=w455:errorcluster)  [unwired: 1 in, 1 out]
              }
              frame True {
                n196 = property on="Enter Manual Mode" class="Bool (strict)"(error in=w459, "Val(Sgnl)"=w460) -> (error out=w458:errorcluster)  [unwired: 1 in, 1 out]
              }
            }
          }
        }
      }
      event "Predict fiducials": Value Change {
        n197 = event-data() -> ()  [unwired: 1 in, 6 out]
        n198 = property on="Predict fiducials" class="Bool (strict)"("Value"=FALSE ("Predict fiducials")) -> ()  [unwired: 2 in, 2 out]
        n199 = call "Predict Fiducials.vi"("input cluster"=w464) -> ("output cluster"=w463:T7)  [unwired: 10 in]
        n200 = property on="Manual Mode On" class="Bool (strict)"() -> ("Value"=w466:bool)  [unwired: 2 in, 2 out]
        n201 = Unbundle By Name(w463) -> ("New Fiducials"=w465:dbl[], "Past Fiducials"=→"predicted fiducials":dbl[][])
        n202 = case shown="False" w466 {
          selector: w466 -> [_ w485]
          tunnel: w465 -> [w469 _]
          frame False {
            n203 = Search 1D Array(1D array=w469, element=0.0) -> (index of element=w473:i32)  [unwired: 1 in]
            n204 = Divide(x=w473, y=3) -> (x/y=w471:dbl)
            n205 = case shown="1" w471 {
              tunnel: TRUE ("Value (Signaling)") -> [w475 w476 w483 w484]
              tunnel: w469 -> [_ w479 _ _]
              frame 0, Default {
                n206 = property on="Go to CH1/FD1" class="Bool (strict)"("Val(Sgnl)"=w475) -> ()  [unwired: 2 in, 2 out]
              }
              frame 1 {
                n207 = Index Array(array=w479, index=6) -> (element=w480:dbl)
                n208 = Not Equal To 0?(x=w480) -> (x != 0?=w477:bool)
                n209 = case shown="True" w477 {
                  tunnel: w476 -> [w481 w482]
                  frame False {
                    n210 = property on="Go to CH8/FD2" class="Bool (strict)"("Val(Sgnl)"=w481) -> ()  [unwired: 2 in, 2 out]
                  }
                  frame True {
                    n211 = property on="Go to CH191/FD5" class="Bool (strict)"("Val(Sgnl)"=w482) -> ()  [unwired: 2 in, 2 out]
                  }
                }
              }
              frame 2 {
                n212 = property on="Go to CH8/FD2" class="Bool (strict)"("Val(Sgnl)"=w483) -> ()  [unwired: 2 in, 2 out]
              }
              frame 3 {
                n213 = property on="Go to CH197/FD4" class="Bool (strict)"("Val(Sgnl)"=w484) -> ()  [unwired: 2 in, 2 out]
              }
            }
          }
          frame True {
            n214 = property on="Enter Manual Mode" class="Bool (strict)"("Val(Sgnl)"=w485) -> ()  [unwired: 2 in, 2 out]
          }
        }
      }
      event "Joystick": Value Change {
        n215 = event-data() -> ()  [unwired: 1 in, 6 out]
        n216 = call "Joystick.vi"("error in (no error)"=w487, "Joystick"="Joystick", "Gantry In"=w490) -> ("error out"=w486:errorcluster, "Gantry Out"=w488:refnum<k24>)  [unwired: 7 in]
      }
      event "Go to Center": Value Change {
        n217 = event-data() -> ()  [unwired: 1 in, 6 out]
        n218 = disable-structure shown="Enabled" {
          disable-tunnel: w498 -> [w502 w517]
          disable-tunnel: [w501 w514] -> w497
          disable-tunnel: w494 -> [_ w515]
          disable-tunnel: [_ w513] -> w493
          frame Disabled {
            n219 = control-ref of="Joystick"() -> (w503:refnum<vi>)
            n220 = property class="Bool (strict)"(reference=w503) -> (reference out=w504:refnum<vi>, "Value"=w505:bool)  [unwired: 1 in, 1 out]
            n221 = case shown="True" w505 {
              selector: w505 -> [_ w512]
              tunnel: w502 -> [w506 w509]
              tunnel: [w506 w508] -> w501
              tunnel: w504 -> [_ w511]
              frame False {
              }
              frame True {
                n222 = Not(x=w512) -> (.not. x?=w507:bool)
                n223 = call "Joystick.vi"("Joystick"=w507, "Gantry In"=w509) -> ("error out"=w510:errorcluster, "Gantry Out"=w508:refnum<k24>)  [unwired: 8 in]
                n224 = property class="Bool (strict)"(reference=w511, error in=w510, "Value"=w507) -> ()  [unwired: 2 out]
              }
            }
          }
          frame Enabled {
            n225 = call "Joystick.vi"("error in (no error)"=w515, "Joystick"=FALSE, "Gantry In"=w517) -> ("error out"=w513:errorcluster, "Gantry Out"=w514:refnum<k24>)  [unwired: 7 in]
          }
        }
        n226 = Unbundle By Name(w499) -> ("XYZTheta"=w500:dbl[])
        n227 = flat-sequence {
          tunnel: w500 -> [w523]
          tunnel: w497 -> [w522]
          tunnel: [w521] -> w495
          tunnel: [w528] -> w496
          tunnel: w495 -> [w528]
          tunnel: w493 -> [w526]
          tunnel: [w524] -> w492
          frame #0 {
            w520 = T8."Disabled and Grayed Out" ("Disabled")
            n228 = call "ClearXYZTheta Go.vi"("Speed"=300.0, "XYZTheta In"=w523, "Gantry In"=w522) -> ("Gantry Out"=w521:refnum<k24>)  [unwired: 6 in, 2 out]
            n229 = property on="Record CH191/FD5" class="Bool (strict)"("DisabledEnum"=w520) -> ()  [unwired: 2 in, 2 out]
            n230 = property on="Go to CH1/FD1" class="Bool (strict)"("DisabledEnum"=w520) -> ()  [unwired: 2 in, 2 out]
            n231 = property on="Go to CH191/FD5" class="Bool (strict)"("DisabledEnum"=w520) -> ()  [unwired: 2 in, 2 out]
            n232 = property on="Go to CH1" class="Bool (strict)"("DisabledEnum"=w520) -> ()  [unwired: 2 in, 2 out]
            n233 = property on="Record CH8/FD2" class="Bool (strict)"("DisabledEnum"=w520) -> ()  [unwired: 2 in, 2 out]
            n234 = property on="Stop Program" class="Bool"("DisabledEnum"=w520) -> ()  [unwired: 2 in, 2 out]
            n235 = property on="Go to CH197/FD4" class="Bool (strict)"("DisabledEnum"=w520) -> ()  [unwired: 2 in, 2 out]
            n236 = property on="Go to CH8/FD2" class="Bool (strict)"("DisabledEnum"=w520) -> ()  [unwired: 2 in, 2 out]
            n237 = property on="Go to Sensor ID" class="Bool (strict)"("DisabledEnum"=w520) -> ()  [unwired: 2 in, 2 out]
            n238 = property on="Record CH1/FD1" class="Bool (strict)"("DisabledEnum"=w520) -> ()  [unwired: 2 in, 2 out]
            n239 = property on="Go to Center" class="Bool"("DisabledEnum"=w520) -> ()  [unwired: 2 in, 2 out]
            n240 = property on="Record CH197/FD4" class="Bool (strict)"("DisabledEnum"=w520) -> ()  [unwired: 2 in, 2 out]
            n241 = shared-variable ".\\Component Tray.lvclass\\Instructions"("Moving to component center. Wait for movement to stop." ("Value (Signaling)")) -> ()  [unwired: 1 in, 1 out]
          }
          frame #1 {
            n242 = property on="Manual Mode On" class="Bool (strict)"(error in=w526) -> (error out=w525:errorcluster, "Value"=w527:bool)  [unwired: 1 in, 1 out]
            n243 = case shown="False" w527 {
              selector: w527 -> [_ w532]
              tunnel: w525 -> [w529 w531]
              tunnel: [w529 w530] -> w524
              frame False {
              }
              frame True {
                n244 = property on="Enter Manual Mode" class="Bool (strict)"(error in=w531, "Val(Sgnl)"=w532) -> (error out=w530:errorcluster)  [unwired: 1 in, 1 out]
              }
            }
          }
        }
      }
      event "Go to CH1": Value Change {
        n245 = event-data() -> ()  [unwired: 1 in, 6 out]
        n246 = property on="Go to CH1" class="Bool (strict)"(error in=w537, "Value"=FALSE ("Go to CH1")) -> (error out=w538:errorcluster)  [unwired: 1 in, 1 out]
        n247 = disable-structure shown="Enabled" {
          disable-tunnel: w547 -> [w549 w564]
          disable-tunnel: [w548 w563] -> w546
          disable-tunnel: w538 -> [_ w561]
          disable-tunnel: [_ w560] -> w536
          frame Disabled {
            n248 = control-ref of="Joystick"() -> (w550:refnum<vi>)
            n249 = property class="Bool (strict)"(reference=w550) -> (reference out=w551:refnum<vi>, "Value"=w552:bool)  [unwired: 1 in, 1 out]
            n250 = case shown="True" w552 {
              selector: w552 -> [_ w559]
              tunnel: w549 -> [w553 w556]
              tunnel: [w553 w555] -> w548
              tunnel: w551 -> [_ w558]
              frame False {
              }
              frame True {
                n251 = Not(x=w559) -> (.not. x?=w554:bool)
                n252 = call "Joystick.vi"("Joystick"=w554, "Gantry In"=w556) -> ("error out"=w557:errorcluster, "Gantry Out"=w555:refnum<k24>)  [unwired: 8 in]
                n253 = property class="Bool (strict)"(reference=w558, error in=w557, "Value"=w554) -> ()  [unwired: 2 out]
              }
            }
          }
          frame Enabled {
            n254 = call "Joystick.vi"("error in (no error)"=w561, "Joystick"=FALSE, "Gantry In"=w564) -> ("error out"=w560:errorcluster, "Gantry Out"=w563:refnum<k24>)  [unwired: 7 in]
          }
        }
        n255 = flat-sequence {
          tunnel: w546 -> [w576]
          tunnel: [w575] -> w543
          tunnel: w541 -> [w573]
          tunnel: [w565] -> w540
          tunnel: w536 -> [w570]
          tunnel: [w569] -> w533
          tunnel: w543 -> [w602]
          tunnel: [w602] -> w542
          tunnel: w540 -> [w600]
          tunnel: [w599] -> w539
          tunnel: [w598] -> w534
          tunnel: w533 -> [w598]
          tunnel: [w608] -> w545
          tunnel: w542 -> [w608]
          tunnel: w539 -> [w606]
          tunnel: [w605] -> w535
          tunnel: w534 -> [w604]
          frame #0 {
            w574 = T8."Disabled and Grayed Out" ("Disabled")
            n256 = Unbundle By Name(w573) -> ("CH1 check"=w568:T4, "CH1 Location"=w571:dbl[], "Protomodule?"=w569:bool)
            n257 = property on="Record CH191/FD5" class="Bool (strict)"("DisabledEnum"=w574) -> ()  [unwired: 2 in, 2 out]
            n258 = property on="Stop Program" class="Bool"("DisabledEnum"=w574) -> ()  [unwired: 2 in, 2 out]
            n259 = property on="Go to CH1/FD1" class="Bool (strict)"("DisabledEnum"=w574) -> ()  [unwired: 2 in, 2 out]
            n260 = property on="Go to CH1" class="Bool (strict)"("DisabledEnum"=w574) -> ()  [unwired: 2 in, 2 out]
            n261 = property on="Record CH1/FD1" class="Bool (strict)"("DisabledEnum"=w574) -> ()  [unwired: 2 in, 2 out]
            n262 = property on="Go to Center" class="Bool"("DisabledEnum"=w574) -> ()  [unwired: 2 in, 2 out]
            n263 = property on="Go to CH191/FD5" class="Bool (strict)"("DisabledEnum"=w574) -> ()  [unwired: 2 in, 2 out]
            n264 = property on="Go to Sensor ID" class="Bool (strict)"("DisabledEnum"=w574) -> ()  [unwired: 2 in, 2 out]
            n265 = property on="Go to CH197/FD4" class="Bool (strict)"("DisabledEnum"=w574) -> ()  [unwired: 2 in, 2 out]
            n266 = property on="Record CH197/FD4" class="Bool (strict)"("DisabledEnum"=w574) -> ()  [unwired: 2 in, 2 out]
            n267 = property on="Go to CH8/FD2" class="Bool (strict)"("DisabledEnum"=w574) -> ()  [unwired: 2 in, 2 out]
            n268 = property on="Record CH8/FD2" class="Bool (strict)"("DisabledEnum"=w574) -> ()  [unwired: 2 in, 2 out]
            n269 = shared-variable ".\\Component Tray.lvclass\\Instructions"("Moving to CH1. Wait for movement to stop." ("Value (Signaling)"), error in=w570) -> (error out=w567:errorcluster)
            n270 = disable-structure shown="Enabled" {
              disable-tunnel: w576 -> [w582 w597]
              disable-tunnel: [w581 w593] -> w575
              disable-tunnel: w567 -> [w580 w595]
              disable-tunnel: w571 -> [w578 w591]
              disable-tunnel: [_ w583] -> w566
              frame Disabled {
                n271 = call "ClearXYZTheta Go.vi"("error in (no error)"=w580, "Speed"=300.0, "XYZTheta In"=w578, "Gantry In"=w582) -> ("error out"=w579:errorcluster, "Gantry Out"=w581:refnum<k24>)  [unwired: 5 in, 1 out]
              }
              frame Enabled {
                w584 = FALSE ("Increment?")
                n272 = Delete From Array(array=w591, length=1, index=2) -> (deleted portion=w587:dbl[], array with subset deleted=w588:dbl[])
                n273 = Index Array(array=w587) -> (element=w586:dbl)  [unwired: 1 in]
                n274 = call "XY Go.vi"("Increment?"=w584, "error in (no error)"=w595, "Speed"=100.0, "XY In"=w588, "Gantry In"=w597) -> ("error out"=w592:errorcluster, "Gantry Out"=w594:refnum<k24>)  [unwired: 4 in, 1 out]
                n275 = call "Z Go.vi"("Increment"=w584, "error in (no error)"=w592, "Speed In"=10.0, "Position In"=w586, "Gantry In"=w594) -> ("error out"=w583:errorcluster, "Gantry Out"=w593:refnum<k24>)  [unwired: 3 in, 2 out]
              }
            }
            n276 = shared-variable ".\\Component Tray.lvclass\\Machine Vision"(w568, error in=w566) -> (error out=w565:errorcluster)
          }
          frame #1 {
            n277 = case shown="True" w598 {
              frame False {
              }
              frame True {
                n278 = Wait (ms)(milliseconds to wait=u32 3000) -> ()  [unwired: 1 out]
              }
            }
            n279 = shared-variable ".\\Component Tray.lvclass\\Instructions"("Checking for CH1." ("Instructions"), error in=w600) -> (error out=w599:errorcluster)
          }
          frame #2 {
            n280 = case shown="False" w604 {
              tunnel: [w611 w624] -> w607
              tunnel: w606 -> [w610 w623]
              tunnel: [w609 w621] -> w605
              frame False {
                n281 = Two Button Dialog(message="Is \"1\" visible on the screen?", 1:"No" ("F button name (\"Cancel\")"), 2:"Yes" ("T button name (\"OK\")")) -> (T button?=w611:bool)
                n282 = case shown="True" w611 {
                  selector: w611 -> [_ w620]
                  tunnel: w610 -> [w616 w618]
                  tunnel: [w615 w619] -> w609
                  frame False {
                    n283 = property on="Enter Manual Mode" class="Bool (strict)"(error in=w616, "Val(Sgnl)"=TRUE ("Value (Signaling)")) -> (error out=w615:errorcluster)  [unwired: 1 in, 1 out]
                  }
                  frame True {
                    n284 = property on="Go to Sensor ID" class="Bool (strict)"(error in=w618, "Val(Sgnl)"=w620) -> (error out=w619:errorcluster)  [unwired: 1 in, 1 out]
                  }
                }
              }
              frame True {
                n285 = shared-variable ".\\Component Tray.lvclass\\Match found?"(error in=w623) -> (w625:bool, error out=w622:errorcluster)
                n286 = case shown="False" w625 {
                  selector: w625 -> [_ w657]
                  tunnel: [w630 w657] -> w624
                  tunnel: w622 -> [w628 w653]
                  tunnel: [w626 w654] -> w621
                  frame False {
                    n287 = shared-variable ".\\Component Tray.lvclass\\Instructions"("Answer prompts." ("Instructions"), error in=w628) -> (error out=w627:errorcluster)
                    n288 = Two Button Dialog(message="Warning: CH1 was not detected automatically.\nIs \"1\" visible on the screen?", 1:"No" ("F button name (\"Cancel\")"), 2:"Yes" ("T button name (\"OK\")")) -> (T button?=w631:bool)
                    n289 = case shown="False" w631 {
                      selector: w631 -> [w639 w651]
                      tunnel: [w639 w651] -> w630
                      tunnel: w627 -> [w636 w650]
                      tunnel: [w635 w649] -> w626
                      frame False {
                        n290 = Two Button Dialog(message="FInd fiducials manually with joystick or restart the automated program?", 1:"Automatic" ("F button name (\"Cancel\")"), 2:"Manual" ("T button name (\"OK\")")) -> (T button?=w638:bool)
                        n291 = case shown="True" w638 {
                          tunnel: TRUE ("Value (Signaling)") -> [w645 w648]
                          tunnel: w636 -> [w644 w647]
                          tunnel: [w643 w646] -> w635
                          frame False {
                            n292 = property on="Go to CH1/FD1" class="Bool (strict)"(error in=w644, "Val(Sgnl)"=w645) -> (error out=w643:errorcluster)  [unwired: 1 in, 1 out]
                          }
                          frame True {
                            n293 = property on="Enter Manual Mode" class="Bool (strict)"(error in=w647, "Val(Sgnl)"=w648) -> (error out=w646:errorcluster)  [unwired: 1 in, 1 out]
                          }
                        }
                      }
                      frame True {
                        n294 = property on="Go to Sensor ID" class="Bool (strict)"(error in=w650, "Val(Sgnl)"=w651) -> (error out=w649:errorcluster)  [unwired: 1 in, 1 out]
                      }
                    }
                  }
                  frame True {
                    n295 = shared-variable ".\\Component Tray.lvclass\\Instructions"("CH1 automatically detected." ("Instructions"), error in=w653) -> (error out=w652:errorcluster)
                    n296 = property on="Manual Mode On" class="Bool (strict)"(error in=w652) -> (error out=w655:errorcluster, "Value"=w658:bool)  [unwired: 1 in, 1 out]
                    n297 = case shown="True" w658 {
                      selector: w658 -> [_ w664]
                      tunnel: w655 -> [w660 w663]
                      tunnel: [w659 w662] -> w654
                      frame False {
                        n298 = property on="Go to Sensor ID" class="Bool (strict)"(error in=w660, "Val(Sgnl)"=TRUE ("Go to Sensor ID")) -> (error out=w659:errorcluster)  [unwired: 1 in, 1 out]
                      }
                      frame True {
                        n299 = property on="Enter Manual Mode" class="Bool (strict)"(error in=w663, "Val(Sgnl)"=w664) -> (error out=w662:errorcluster)  [unwired: 1 in, 1 out]
                      }
                    }
                  }
                }
              }
            }
            "CH1 correct?" <- w607
          }
        }
      }
      event "Enter Manual Mode": Value Change {
        w673 = T8."Enabled" ("Disabled")
        n300 = event-data() -> ()  [unwired: 1 in, 6 out]
        n301 = Unbundle By Name(w669) -> ("4 fiducials?"=w668:bool)
        n302 = case shown="True" w668 {
          tunnel: [T8."Disabled and Grayed Out" ("Disabled") T8."Enabled" ("Disabled")] -> w672
          frame False {
          }
          frame True {
          }
        }
        n303 = property on="Enter Manual Mode" class="Bool (strict)"("Value"=FALSE ("Enter Manual Mode")) -> ()  [unwired: 2 in, 2 out]
        n304 = local read "Enter Manual Mode"() -> (w665:bool)
        n305 = property on="Go to CH1" class="Bool (strict)"("DisabledEnum"=w673) -> ()  [unwired: 2 in, 2 out]
        n306 = case shown="True" w665 {
          selector: w665 -> [_ w674]
          frame False {
          }
          frame True {
            "Manual Mode On" <- w674
          }
        }
        n307 = shared-variable ".\\Component Tray.lvclass\\Instructions"("Now in manual mode." ("Value (Signaling)")) -> ()  [unwired: 1 in, 1 out]
        n308 = property on="Go to Sensor ID" class="Bool (strict)"("DisabledEnum"=w673) -> ()  [unwired: 2 in, 2 out]
        n309 = property on="Record CH1/FD1" class="Bool (strict)"("DisabledEnum"=w673) -> ()  [unwired: 2 in, 2 out]
        n310 = property on="Go to CH8/FD2" class="Bool (strict)"("DisabledEnum"=w673) -> ()  [unwired: 2 in, 2 out]
        n311 = property on="Go to Center" class="Bool"("DisabledEnum"=w673) -> ()  [unwired: 2 in, 2 out]
        n312 = property on="Record CH8/FD2" class="Bool (strict)"("DisabledEnum"=w673) -> ()  [unwired: 2 in, 2 out]
        n313 = property on="Go to CH1/FD1" class="Bool (strict)"("DisabledEnum"=w673) -> ()  [unwired: 2 in, 2 out]
        n314 = property on="Stop Program" class="Bool"("DisabledEnum"=w673) -> ()  [unwired: 2 in, 2 out]
        n315 = property on="Record CH197/FD4" class="Bool (strict)"("DisabledEnum"=w672) -> ()  [unwired: 2 in, 2 out]
        n316 = property on="Record CH191/FD5" class="Bool (strict)"("DisabledEnum"=w672) -> ()  [unwired: 2 in, 2 out]
        n317 = property on="Go to CH197/FD4" class="Bool (strict)"("DisabledEnum"=w672) -> ()  [unwired: 2 in, 2 out]
        n318 = property on="Go to CH191/FD5" class="Bool (strict)"("DisabledEnum"=w672) -> ()  [unwired: 2 in, 2 out]
      }
      event "Go to Sensor ID": Value Change {
        n319 = event-data() -> ()  [unwired: 1 in, 6 out]
        n320 = flat-sequence {
          tunnel: w685 -> [w691]
          tunnel: w688 -> [w692]
          tunnel: w689 -> [w693]
          tunnel: [w693] -> w682
          tunnel: [w692] -> w680
          tunnel: [w691] -> w678
          tunnel: ["Go to Sensor ID"] -> w683
          tunnel: w682 -> [w698]
          tunnel: [w698] -> w681
          tunnel: w680 -> [w697]
          tunnel: [w697] -> w679
          tunnel: w678 -> [w695]
          tunnel: [w694] -> w677
          tunnel: [w703] -> w686
          tunnel: [w699] -> w684
          tunnel: w681 -> [w702]
          tunnel: w679 -> [w704]
          tunnel: w677 -> [w700]
          tunnel: [w1025] -> w687
          tunnel: w686 -> [w1025]
          frame #0 {
          }
          frame #1 {
            n321 = property on="Go to Sensor ID" class="Bool (strict)"(error in=w695, "Value"=FALSE ("Go to Sensor ID")) -> (error out=w694:errorcluster)  [unwired: 1 in, 1 out]
          }
          frame #2 {
            n322 = Unbundle By Name(w702) -> ("Protomodule?"=w701:bool)
            n323 = case shown="True" w701 {
              tunnel: w702 -> [_ w743]
              tunnel: w704 -> [w706 w713]
              tunnel: [w706 w742] -> w703
              tunnel: w700 -> [w705 w710]
              tunnel: [w705 w720] -> w699
              frame False {
              }
              frame True {
                w722 = T8."Disabled and Grayed Out" ("Disabled")
                # "Will replace this with automatic checking"
                n324 = Unbundle By Name(w743) -> ("Sensor ID Location"=w741:dbl[], "XYZTheta"=w740:dbl[], "Position"=w739:i32, "Pos multiplier"=w717:dbl)
                n325 = Multiply(x=-0.44 ("r"), y=w717) -> (x*y=w718:dbl)
                n326 = Index Array(array=w740, index=3) -> (element=w730:dbl)
                n327 = local read "CH197/FD4 XYZ"() -> (w716:dbl[])
                n328 = Array Subset(array=w741, length=2) -> (w731:dbl[])  [unwired: 1 in]
                n329 = Add(x=w730, y=1.5707963267948966) -> (x+y=w735:dbl)
                n330 = local write "Machine Vision"(Machine_Vision."sensor edge init" ("Machine Vision")) -> ()
                n331 = Index Array(array=w716, index=2) -> (element=w714:dbl)
                n332 = for {
                  N: 5 -> [_]
                  shift-right: [w1007] -> _
                  shift-left: w731 -> [w1011]
                  shift-right: [w1010] -> _
                  shift-left: w735 -> [w1010]
                  tunnel: [w1007] -> w734 mode=indexing
                  shift-right: [w1006] -> _
                  shift-left: w718 -> [w1006]
                  n333 = in-place {
                    in-place-border: w1010 -> [w1013]
                    in-place-border: [w1013] -> _
                    in-place-border: w1006 -> [w1012]
                    n334 = in-place-array #2(w1011, 0, 1) -> (w1019:dbl, w1018:dbl)
                    n335 = Polar To Re/Im(2:w1013, 3:w1012) -> (0:w1016:dbl, 1:w1017:dbl)
                    n336 = Add(x=w1019, y=w1017) -> (x+y=w1015:dbl)
                    n337 = Add(x=w1018, y=w1016) -> (x+y=w1014:dbl)
                    n338 = in-place-array #2(w1015, w1014) -> (w1007:dbl[])  [unwired: 2 out]
                  }
                }
                n339 = property on="Go to CH1" class="Bool (strict)"("DisabledEnum"=w722) -> ()  [unwired: 2 in, 2 out]
                n340 = property on="Go to CH1/FD1" class="Bool (strict)"("DisabledEnum"=w722) -> ()  [unwired: 2 in, 2 out]
                n341 = property on="Go to CH191/FD5" class="Bool (strict)"("DisabledEnum"=w722) -> ()  [unwired: 2 in, 2 out]
                n342 = property on="Record CH8/FD2" class="Bool (strict)"("DisabledEnum"=w722) -> ()  [unwired: 2 in, 2 out]
                n343 = property on="Go to CH197/FD4" class="Bool (strict)"("DisabledEnum"=w722) -> ()  [unwired: 2 in, 2 out]
                n344 = property on="Go to CH8/FD2" class="Bool (strict)"("DisabledEnum"=w722) -> ()  [unwired: 2 in, 2 out]
                n345 = property on="Record CH1/FD1" class="Bool (strict)"("DisabledEnum"=w722) -> ()  [unwired: 2 in, 2 out]
                n346 = property on="Record CH191/FD5" class="Bool (strict)"("DisabledEnum"=w722) -> ()  [unwired: 2 in, 2 out]
                n347 = property on="Go to Center" class="Bool"("DisabledEnum"=w722) -> ()  [unwired: 2 in, 2 out]
                n348 = property on="Go to Sensor ID" class="Bool (strict)"("DisabledEnum"=w722) -> ()  [unwired: 2 in, 2 out]
                n349 = property on="Record CH197/FD4" class="Bool (strict)"("DisabledEnum"=w722) -> ()  [unwired: 2 in, 2 out]
                n350 = property on="Stop Program" class="Bool"("DisabledEnum"=w722) -> ()  [unwired: 2 in, 2 out]
                n351 = call "Z Go.vi"("error in (no error)"=w710, "Speed In"=5.0, "Position In"=w714, "Gantry In"=w713) -> ("error out"=w709:errorcluster, "Gantry Out"=w712:refnum<k24>)  [unwired: 4 in, 2 out]
                n352 = shared-variable ".\\Component Tray.lvclass\\Instructions"("Now determining sensor ID. This takes several seconds, please wait." ("Value (Signaling)")) -> ()  [unwired: 1 in, 1 out]
                n353 = Build Array (concatenate)(w731, w734) -> (w732:dbl[][])
                n354 = disable-structure shown="Enabled" {
                  disable-tunnel: [w773 w850 w939] -> w742
                  disable-tunnel: w739 -> [w772 _ _]
                  disable-tunnel: w732 -> [w766 w849 w938]
                  disable-tunnel: w712 -> [w765 w848 w941]
                  disable-tunnel: w730 -> [w749 _ _]
                  disable-tunnel: [w747 _ _] -> w729
                  disable-tunnel: [w746 w834 w929] -> w728
                  disable-tunnel: [w745 w843 w937] -> w720
                  disable-tunnel: w709 -> [w744 w847 w940]
                  disable-tunnel: w717 -> [_ w842 w942]
                  disable-tunnel: [_ w833 w928] -> w708
                  frame Disabled {
                    n355 = call "Base File Path.vi"() -> ("Paths Out"=w771:T14)  [unwired: 11 in]
                    n356 = Unbundle By Name(w771) -> ("Components Folder"=w770:path)
                    n357 = Build Path(base path=w770, name or relative path=path "temp") -> (appended path=w769:path)
                    n358 = Create Folder(path (use dialog)=w769, error in=w744) -> (created path=w768:path, error out=w751:errorcluster)  [unwired: 1 in, 1 out]
                    n359 = for {
                      shift-right: [w788] -> w773
                      shift-left: w765 -> [w789]
                      shift-right: [w786] -> w752
                      shift-left: w768 -> [w786]
                      tunnel: w766 -> [w785] mode=indexing
                      shift-right: [w783] -> w750
                      shift-left: w751 -> [w784]
                      tunnel: [w782] -> w747 mode=indexing
                      i -> [w787]
                      n360 = flat-sequence {
                        tunnel: w789 -> [w796]
                        tunnel: [w793] -> w781
                        tunnel: w785 -> [w792]
                        tunnel: w784 -> [w791]
                        tunnel: [w790] -> w780
                        tunnel: w781 -> [w807]
                        tunnel: [w807] -> w779
                        tunnel: w787 -> [w803]
                        tunnel: w786 -> [w800]
                        tunnel: [w799] -> w778
                        tunnel: [w797] -> w777
                        tunnel: w780 -> [w797]
                        tunnel: w779 -> [w813]
                        tunnel: w778 -> [w809]
                        tunnel: w777 -> [w812]
                        tunnel: [w813] -> w776
                        tunnel: [w811] -> w775
                        tunnel: [w809] -> w774
                        tunnel: [w815] -> w783
                        tunnel: [w818] -> w788
                        tunnel: w776 -> [w818]
                        tunnel: w775 -> [w816]
                        tunnel: w774 -> [w817]
                        tunnel: [w814] -> w782
                        frame #0 {
                          n361 = call "XY Go.vi"("return immediately"=FALSE, "error in (no error)"=w791, "Speed"=100.0, "XY In"=w792, "Gantry In"=w796) -> ("error out"=w790:errorcluster, "Gantry Out"=w793:refnum<k24>)  [unwired: 4 in, 1 out]
                        }
                        frame #1 {
                          n362 = Wait (ms)(milliseconds to wait=u32 1000) -> ()  [unwired: 1 out]
                          n363 = Number To Decimal String(number=w803) -> (decimal integer string=w805:string)  [unwired: 1 in]
                          n364 = Concatenate Strings("temp" ("string"), w805, ".bmp" ("string")) -> (w806:string)
                          n365 = String To Path(string=w806) -> (path=w804:path)
                          n366 = Build Path(base path=w800, name or relative path=w804) -> (appended path=w799:path)
                        }
                        frame #2 {
                          n367 = local read "Image"() -> (w808:T5)
                          n368 = Wait (ms)(milliseconds to wait=u32 1000) -> ()  [unwired: 1 out]
                          n369 = call-poly "IMAQ Write File 2"("error in (no error)"=w812, "File Path"=w809, "Image"=w808) -> ("error out"=w811:errorcluster)  [unwired: 7 in, 1 out]
                        }
                        frame #3 {
                          n370 = disable-structure shown="Enabled" {
                            disable-tunnel: w817 -> [w825 w831]
                            disable-tunnel: w816 -> [w824 w830]
                            disable-tunnel: [w823 w829] -> w815
                            disable-tunnel: [w821 w832] -> w814
                            frame Disabled {
                              n371 = call <vilib>:"Read BMP File.vi"("error in (no error)"=w824, "path to BMP file"=w825) -> ("error out"=w823:errorcluster, "image data"=w820:T15)  [unwired: 7 in, 1 out]
                              n372 = in-place {
                                n373 = in-place-cluster #3(w820) -> ("Rectangle"=w828:T13)
                                n374 = Divide(x=w828, y=T13 {"left"=2, "top"=2, "right"=2, "bottom"=2}) -> (x/y=w826:T16)
                                n375 = in-place-cluster #3("Rectangle"=w826) -> (w819:T15)
                              }
                              n376 = call <vilib>:"Draw Flattened Pixmap.vi"("image data"=w819, "picture"=picture data[5B]) -> ("new picture"=w821:picture)  [unwired: 7 in]
                            }
                            frame Enabled {
                              n377 = call "Resize Image to a Container 2012 NIVerified.vi"("error in (no error)"=w830, "Path to Image (PNG, JPEG, BMP)"=w831) -> ("error out"=w829:errorcluster, "Resized Image"=w832:picture)  [unwired: 7 in]
                            }
                          }
                        }
                      }
                    }
                    n378 = call "Base File Path.vi"() -> ("Paths Out"=w760:T14)  [unwired: 11 in]
                    n379 = Unbundle By Name(w760) -> ("Components Folder"=w759:path)
                    n380 = call "Get Python Version.vi"("error in (no error)"=w750) -> ("Python Version"=w756:string, "error out"=w755:errorcluster)  [unwired: 9 in]
                    n381 = Build Path(base path=w759, name or relative path=path "SensorID.py") -> (appended path=w758:path)
                    n382 = Open Python Session(python version=w756, 3:w755) -> (session out=w764:refnum<k35>, error out=w762:errorcluster)  [unwired: 1 in]
                    n383 = Path To String(path=w752) -> (string=w753:string)
                    n384 = node(w764, w758, "read_sensor_ID" ("function name"), w762, "read_sensor_ID" ("string"), w753, w772, w749) -> (w763:refnum<k35>, w761:errorcluster, w746:string)  [unwired: 3 in, 2 out]
                    n385 = Close Python Session(session in=w763, error in=w761) -> (11:w745:errorcluster)
                  }
                  frame Disabled {
                    n386 = for {
                      shift-right: [w913] -> w850
                      shift-left: w848 -> [w914]
                      tunnel: w849 -> [w912] mode=indexing
                      shift-right: [w910] -> w844
                      shift-left: w847 -> [w911]
                      tunnel: [w905] -> w846 mode=indexing
                      n387 = flat-sequence {
                        tunnel: w914 -> [w921]
                        tunnel: [w918] -> w907
                        tunnel: w912 -> [w917]
                        tunnel: w911 -> [w916]
                        tunnel: [w915] -> w906
                        tunnel: w907 -> [w924]
                        tunnel: w906 -> [w923]
                        tunnel: [w924] -> w909
                        tunnel: [w923] -> w908
                        tunnel: [w926] -> w910
                        tunnel: [w927] -> w913
                        tunnel: w909 -> [w927]
                        tunnel: w908 -> [w926]
                        tunnel: [w925] -> w905
                        frame #0 {
                          n388 = call "XY Go.vi"("return immediately"=FALSE, "error in (no error)"=w916, "Speed"=100.0, "XY In"=w917, "Gantry In"=w921) -> ("error out"=w915:errorcluster, "Gantry Out"=w918:refnum<k24>)  [unwired: 4 in, 1 out]
                        }
                        frame #1 {
                          n389 = Wait (ms)(milliseconds to wait=u32 1000) -> ()  [unwired: 1 out]
                        }
                        frame #2 {
                          n390 = local read "Image"() -> (w925:T5)
                        }
                      }
                    }
                    n391 = for {
                      tunnel: w846 -> [w864] mode=indexing
                      tunnel: T5 refnum ("Template Image") -> [w863]
                      shift-right: [w861] -> w843
                      shift-left: w844 -> [w862]
                      tunnel: w842 -> [w854]
                      tunnel: [w852] -> w835 mode=indexing
                      tunnel: [w851] -> w833 mode=indexing
                      n392 = call "IMAQ Match Pattern 4"("Image"=w864, "Algorithm"="Algorithm", "Template Image"=w863, "ROI Descriptor"="ROI Descriptor", "Parameters"="Parameters", "error in (no error)"=w862, "Advanced Options"="Advanced Options") -> ("Matches (real-world)"=w853:T17, "Number of Matches"=w856:i32, "error out"=w861:errorcluster)  [unwired: 4 in, 2 out]
                      n393 = Greater Than 0?(x=w856) -> (x > 0?=w855:bool)
                      n394 = case shown="False" w855 {
                        tunnel: w854 -> [w868 _]
                        tunnel: [w866 0 ("index")] -> w851
                        tunnel: w853 -> [w865 _]
                        frame False {
                          n395 = for {
                            tunnel: w868 -> [w877]
                            tunnel: [w876] -> w867 mode=indexing
                            tunnel: w865 -> [w871] mode=indexing
                            n396 = Unbundle By Name(w871) -> ("Position"=w870:cluster{"x":sgl, "y":sgl})
                            n397 = Cluster To Array(cluster=w870) -> (array=w869:sgl[])
                            n398 = Index Array(array=w869, index #1=0 ("index"), index #2=1 ("index")) -> (element #2=w878:sgl)  [unwired: 1 out]
                            n399 = Multiply(x=w878, y=w877) -> (x*y=w874:dbl)
                            n400 = Absolute Value(x=w874) -> (abs(x)=w873:dbl)
                            n401 = Greater?(x=w873, y=0.25) -> (0:w872:bool)
                            n402 = case shown="False" w872 {
                              tunnel: w874 -> [w882 _]
                              tunnel: [w881 0 ("index")] -> w876
                              frame False {
                                n403 = Greater?(x=w882, y=0.1) -> (0:w884:bool)
                                n404 = case shown="False" w884 {
                                tunnel: w882 -> [w886 _]
                                tunnel: [w885 8 ("index")] -> w881
                                frame False {
                                n405 = Greater?(x=w886, y=0.01) -> (0:w888:bool)
                                n406 = case shown="False" w888 {
                                tunnel: w886 -> [w893 _]
                                tunnel: [w890 4 ("index")] -> w885
                                frame False {
                                n407 = Negate(x=w893) -> (-x=w889:dbl)
                                n408 = Greater?(x=w889, y=0.1) -> (0:w891:bool)
                                n409 = case shown="False" w891 {
                                tunnel: [w894 1 ("index")] -> w890
                                tunnel: w889 -> [w896 _]
                                frame False {
                                n410 = Greater?(x=w896, y=0.01) -> (0:w895:bool)
                                n411 = case shown="True" w895 {
                                tunnel: [0 ("index") 2 ("index")] -> w894
                                frame False {
                                }
                                frame True {
                                }
                                }
                                }
                                frame True {
                                }
                                }
                                }
                                frame True {
                                }
                                }
                                }
                                frame True {
                                }
                                }
                              }
                              frame True {
                              }
                            }
                          }
                          n412 = Add Array Elements(numeric array=w867) -> (sum=w866:i32)
                        }
                        frame True {
                        }
                      }
                      n413 = Number To Decimal String(number=w851) -> (decimal integer string=w852:string)  [unwired: 1 in]
                    }
                    n414 = Index Array(array=w835) -> (element #1=w841:string, element #2=w840:string, element #3=w839:string, element #4=w838:string, element #5=w837:string, element #6=w836:string)  [unwired: 6 in]
                    n415 = Concatenate Strings(w841, w840, w839, w838, w837, w836) -> (w834:string)
                  }
                  frame Enabled {
                    n416 = for {
                      tunnel: w942 -> [w950]
                      shift-right: [w946] -> w939
                      shift-left: w941 -> [w949]
                      shift-right: [w947] -> w937
                      shift-left: w940 -> [w948]
                      tunnel: w938 -> [w945] mode=indexing
                      tunnel: [w944] -> w936 mode=indexing
                      tunnel: [w943] -> w928 mode=indexing
                      n417 = flat-sequence {
                        tunnel: w949 -> [w955]
                        tunnel: [w954] -> w946
                        tunnel: w948 -> [w953]
                        tunnel: [w952] -> w947
                        tunnel: w945 -> [w951]
                        tunnel: w950 -> [w967]
                        tunnel: [w961] -> w943
                        frame #0 {
                          n418 = call "XY Go.vi"("error in (no error)"=w953, "Speed"=100.0, "XY In"=w951, "Gantry In"=w955) -> ("error out"=w952:errorcluster, "Gantry Out"=w954:refnum<k24>)  [unwired: 5 in, 1 out]
                        }
                        frame #1 {
                          n419 = Wait (ms)(milliseconds to wait=u32 500) -> ()  [unwired: 1 out]
                        }
                        frame #2 {
                          n420 = local write "Machine Vision"(Machine_Vision."sensor ID" ("Machine Vision")) -> ()
                        }
                        frame #3 {
                          n421 = Wait (ms)(milliseconds to wait=u32 2000) -> ()  [unwired: 1 out]
                        }
                        frame #4 {
                          n422 = local read "All Matches XY"() -> (w966:sgl[][])
                          n423 = Empty Array?(array=w966) -> (empty?=w965:bool)
                          n424 = Initialize Array(FALSE, 4 ("dimension size")) -> (w964:bool[])
                          n425 = case shown="False" w965 {
                            tunnel: w967 -> [w971 _]
                            tunnel: w966 -> [w970 _]
                            tunnel: w964 -> [w969 w1004]
                            tunnel: [w968 w1004] -> w960
                            frame False {
                              n426 = for {
                                tunnel: w970 -> [w982] mode=indexing
                                tunnel: w971 -> [w978]
                                shift-right: [w972] -> w968
                                shift-left: w969 -> [w973]
                                n427 = Index Array(array=w982, index #1=0 ("index"), index #2=1 ("index")) -> (element #2=w979:sgl)  [unwired: 1 out]
                                n428 = Multiply(x=w979, y=w978) -> (x*y=w976:dbl)
                                n429 = Absolute Value(x=w976) -> (abs(x)=w975:dbl)
                                n430 = Greater?(x=w975, y=0.25) -> (0:w974:bool)
                                n431 = case shown="False" w974 {
                                tunnel: w976 -> [w987 _]
                                tunnel: w973 -> [w986 w1003]
                                tunnel: [w983 w1003] -> w972
                                frame False {
                                n432 = Greater?(x=w987, y=0.1) -> (0:w989:bool)
                                n433 = case shown="False" w989 {
                                tunnel: w987 -> [w991 _]
                                tunnel: [w990 3 ("index")] -> w984
                                frame False {
                                n434 = Greater?(x=w991, y=0.01) -> (0:w993:bool)
                                n435 = case shown="False" w993 {
                                tunnel: w991 -> [w998 _]
                                tunnel: [w995 2 ("index")] -> w990
                                frame False {
                                n436 = Negate(x=w998) -> (-x=w994:dbl)
                                n437 = Greater?(x=w994, y=0.1) -> (0:w996:bool)
                                n438 = case shown="True" w996 {
                                tunnel: [1 ("index") 0 ("index")] -> w995
                                frame False {
                                }
                                frame True {
                                }
                                }
                                }
                                frame True {
                                }
                                }
                                }
                                frame True {
                                }
                                }
                                n439 = Replace Array Subset(array=w986, new element=TRUE ("new element/subarray"), index=w984) -> (w983:bool[])
                                }
                                frame True {
                                }
                                }
                              }
                            }
                            frame True {
                            }
                          }
                          n440 = Boolean Array To Number(Boolean array=w960) -> (number=w961:u32)
                        }
                        frame #5 {
                          n441 = local write "Machine Vision"(Machine_Vision."sensor edge init" ("Machine Vision")) -> ()
                        }
                      }
                      n442 = Number To Decimal String(number=w943) -> (decimal integer string=w944:string)  [unwired: 1 in]
                    }
                    n443 = Index Array(array=w936) -> (element #1=w935:string, element #2=w934:string, element #3=w933:string, element #4=w932:string, element #5=w931:string, element #6=w930:string)  [unwired: 6 in]
                    n444 = Concatenate Strings(w935, w934, w933, w932, w931, w930) -> (w929:string)
                  }
                }
                "Sensor ID" <- w728
                "Sensor ID" <- w729
                "Array" <- w708
                n445 = Concatenate Strings(w728, " is the sensor ID. Does this match the input?" ("string")) -> (w726:string)
                n446 = Two Button Dialog(message=w726, 1:"No" ("F button name (\"Cancel\")"), 2:"Yes" ("T button name (\"OK\")")) -> (T button?=w723:bool)
                n447 = case shown="True" w723 {
                  frame False {
                  }
                  frame True {
                  }
                }
              }
            }
          }
          frame #3 {
            n448 = local write "Checking Sensor ID"(FALSE ("Checking Sensor ID")) -> ()
            n449 = Two Button Dialog(message="Ready to Submit?", 1:"No" ("F button name (\"Cancel\")"), 2:"Yes" ("T button name (\"OK\")")) -> (T button?=w1021:bool)
            n450 = case shown="True" w1021 {
              selector: w1021 -> [_ w1027]
              frame False {
                n451 = property on="Enter Manual Mode" class="Bool (strict)"("Val(Sgnl)"=TRUE ("Value (Signaling)")) -> ()  [unwired: 2 in, 2 out]
              }
              frame True {
                n452 = property on="Auto Submit" class="Bool (strict)"("Val(Sgnl)"=w1027) -> ()  [unwired: 2 in, 2 out]
              }
            }
          }
        }
        "Checking Sensor ID" <- w683
      }
    }
    n453 = Equal?(x=w104, y=0) -> (x = y?=w102:bool)
    n454 = case shown="True" w102 {
      tunnel: w101 -> [_ w122]
      tunnel: w100 -> [_ w114]
      frame False {
      }
      frame True {
        w119 = T8."Disabled and Grayed Out" ("Disabled")
        n455 = Unbundle By Name(w114) -> ("Assembly Type"=w113:string, "Tray Number"=w112:string)
        n456 = property on="Go to CH1" class="Bool (strict)"("DisabledEnum"=w119) -> ()  [unwired: 2 in, 2 out]
        n457 = shared-variable ".\\Component Tray.lvclass\\Machine Vision"(T9."Assembly Tray Circle" ("Machine Vision")) -> ()  [unwired: 1 in, 1 out]
        n458 = Format Into String(format string="%d", initial string="Now measuring Position ", w122) -> (resulting string=w118:string)  [unwired: 1 in, 1 out]
        n459 = property on="Stop Program" class="Bool"("DisabledEnum"=w119) -> ()  [unwired: 2 in, 2 out]
        n460 = property on="Record CH197/FD4" class="Bool (strict)"("DisabledEnum"=w119) -> ()  [unwired: 2 in, 2 out]
        n461 = property on="Go to CH8/FD2" class="Bool (strict)"("DisabledEnum"=w119) -> ()  [unwired: 2 in, 2 out]
        n462 = property on="Record CH8/FD2" class="Bool (strict)"("DisabledEnum"=w119) -> ()  [unwired: 2 in, 2 out]
        n463 = property on="Record CH1/FD1" class="Bool (strict)"("DisabledEnum"=w119) -> ()  [unwired: 2 in, 2 out]
        n464 = property on="Go to CH197/FD4" class="Bool (strict)"("DisabledEnum"=w119) -> ()  [unwired: 2 in, 2 out]
        n465 = property on="Go to CH191/FD5" class="Bool (strict)"("DisabledEnum"=w119) -> ()  [unwired: 2 in, 2 out]
        n466 = property on="Go to Center" class="Bool"("DisabledEnum"=w119) -> ()  [unwired: 2 in, 2 out]
        n467 = property on="Go to Sensor ID" class="Bool (strict)"("DisabledEnum"=w119) -> ()  [unwired: 2 in, 2 out]
        n468 = property on="Record CH191/FD5" class="Bool (strict)"("DisabledEnum"=w119) -> ()  [unwired: 2 in, 2 out]
        n469 = property on="Go to CH1/FD1" class="Bool (strict)"("DisabledEnum"=w119) -> ()  [unwired: 2 in, 2 out]
        n470 = shared-variable ".\\Component Tray.lvclass\\Instructions"("Answer prompts then wait for gantry movement." ("Instructions")) -> (error out=w111:errorcluster)  [unwired: 1 in]
        n471 = Concatenate Strings(w118, " on Tray " ("string"), w112, " for " ("string"), w113) -> (→"Tray and Position":string)
        n472 = property on="Go to CH1/FD1" class="Bool (strict)"(error in=w111, "Val(Sgnl)"=TRUE ("Value (Signaling)")) -> ()  [unwired: 1 in, 2 out]
      }
    }
  }
  "Gantry Out" <- w14
